vi "ConvertGoop2ToGoop3.vi"() -> (0 "error out":errorcluster)   [LabVIEW 2014]
uses:
  <resource>/Framework/Providers/Open_GDS/ClassProviders/Common/ConvertGoop2ToGoop3_SubVIs/ConvertGoop2ToGoop3_ClassInfo.ctl
  <resource>/Framework/Providers/Open_GDS/ClassProviders/Common/LvClass_class/GDSLvCLass_ClassSettingsType.ctl
  <resource>/Framework/Providers/Open_GDS/ClassProviders/Common/LvClass_class/GDSLvClass_PlugIn.ctl
  <resource>/Framework/Providers/Open_GDS/ClassProviders/Common/LvClass_class/GDSLvClass_PlugInTypes.ctl
  <vilib>/Utility/miscctls.llb/LVPositionTypeDef.ctl
  <vilib>/Utility/error.llb/DialogType.ctl
  <vilib>/picture/picture.llb/imagedata.ctl
  <resource>/Framework/Providers/Open_GDS/ClassProviders/Provider_EndevoGOOP300/Templates/EndevoTemplateNames.ctl
  <resource>/Framework/Providers/Open_GDS/ClassProviders/Provider_EndevoGOOP300/EndevoProviderName.ctl
  <vilib>/regexp/Match Regular Expression.xnode
panel:
  in  "Cancel":bool
  in  "Next":bool
  out "Tab":T1(tab)
  in  "Current GOOP2 top directory":path
  out "Additional VIs that has been found\nand will be relinked:":i32
  out "GOOP2 classes found":string
  in  "VisToRelink":path[](array[path])
  in  "Project":path caption="This project will be created and have all classes added to it:"
  in  "Progress":i32(listbox)
  in  "Done":bool
  out "State":string
  # "1."
  # "Select Top folder to start a recursive search for GOOP2 classes and application VIs."
  # "2."
  # "These classes\nhave been found.\n\nDo you want to convert them?"
  # "3."
  # "Have you backed up all your VIs in the selected folder?"
  # "Have you checked that all files in\nthe selected folder are writeable?"
  # "Relinking VIs outside top folder?\nIf you want to relink any VIs to the new classes that are outside the selected top folder, add them to the list below"
  # "4."
  # "Save VI dialog boxes!?!\nIt might pop up dialog boxes that asks you to save VIs that will be unloaded from memory, JUST press cancel for those."
  # "5."
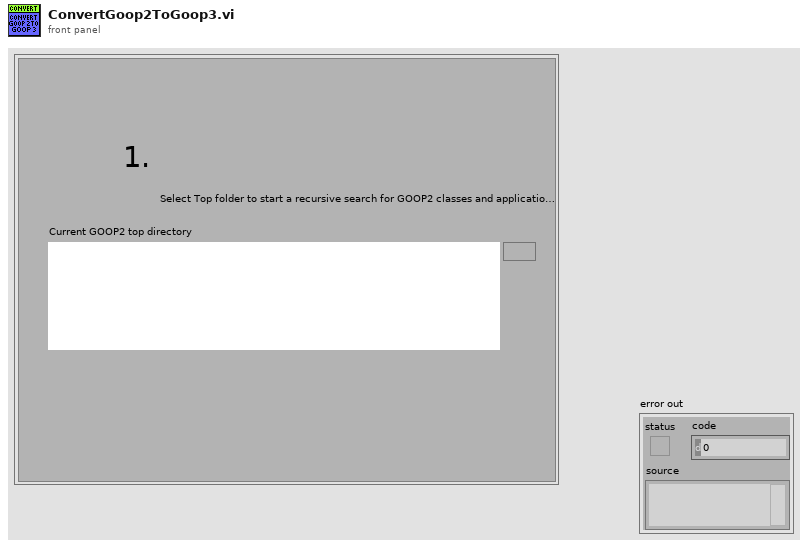
[diagram p1: front panel]
types:
  T1 = enum32{"GOOP2Dir", "ClassesFound", "BackedUp", "Start?", "Converting"}
  T2 = typedef "ConvertGoop2ToGoop3_ClassInfo.ctl" = cluster{"NoOfInheritance":i32, "LvClassPath":path, "ClassName":string, "ClassPrefix":string, "IsLLB":bool, "ClassFolder":path, "ViRefs":refnum<vi>[], "ClassRef":refnum<vi>, "InheritsFrom":path, "RootClass":path, "ViPathes":path[], "AllInheritanceClasses":string[], "TemplateVersionUsed":string, "UsingClassAttributes":bool, "ClassSettings":T3, "HeaderIcon":u8[][]}
  T3 = typedef "GDSLvCLass_ClassSettingsType.ctl" = cluster{"ClassProviderName":string, "ClassTemplateUsed":string, "ClassTemplateVersion":string, "ClassDescription":string, "PlugIns":T4[], "ConnectorPanePattern":string}
  T4 = typedef "GDSLvClass_PlugIn.ctl" = cluster{"Type":T5, "ID":string, "Version":string, "Path":path, "Name":string, "Data":variant}
  T5 = typedef "GDSLvClass_PlugInTypes.ctl" = enum16{"DesignPattern", "MethodTypes"}
  T6 = typedef "LVPositionTypeDef.ctl" = cluster{"Left":i32, "Top":i32}
  T7 = cluster{"TopFolderPath":path, "Classes":T2[], "SetToDynamicDispatch":refnum<vi>[], "error":errorcluster, "Project":path, "ProjectRef":refnum<vi>, "My Computer":refnum<vi>, "AppRef":refnum<vi>, "VIsToRelink":refnum<vi>[], "VIsToRelink(Paths)":path[], "CallParentMethod":cluster{"VIRef":refnum<vi>, "Position":T6}[], "TemplateVersionUsed":string}
  T8 = enum32{"GOOP2Dir", "ClassesFound", "GOOP3Dir", "Start?", "Converting"}
  T9 = typedef "imagedata.ctl" = cluster{"image type":i32, "image depth":i32, "image":u8[], "mask":u8[], "colors":u32[], "Rectangle":cluster{"left":i16, "top":i16, "right":i16, "bottom":i16}}
  T10 = typedef "EndevoTemplateNames.ctl" = enum16{"BaseTemplate", "SubTemplate", "BaseTemplate_4x4x4", "SubTemplate_4x4x4", "SingletonTemplate"}
  T11 = typedef "EndevoProviderName.ctl" = enum16{"EndevoGOOP300"}
  T12 = typedef "DialogType.ctl" = u16
  T13 = enum32{"invalid VI type", "Standard VI", "Control VI", "Global VI", "Polymorphic VI", "Configuration VI", "SubSystem", "Facade VI", "Method VI", "Statechart Diagram VI"}
  T14 = enum16{"Invalid Wire Rule", "Required", "Recommended", "Optional", "Dynamic Dispatch"}
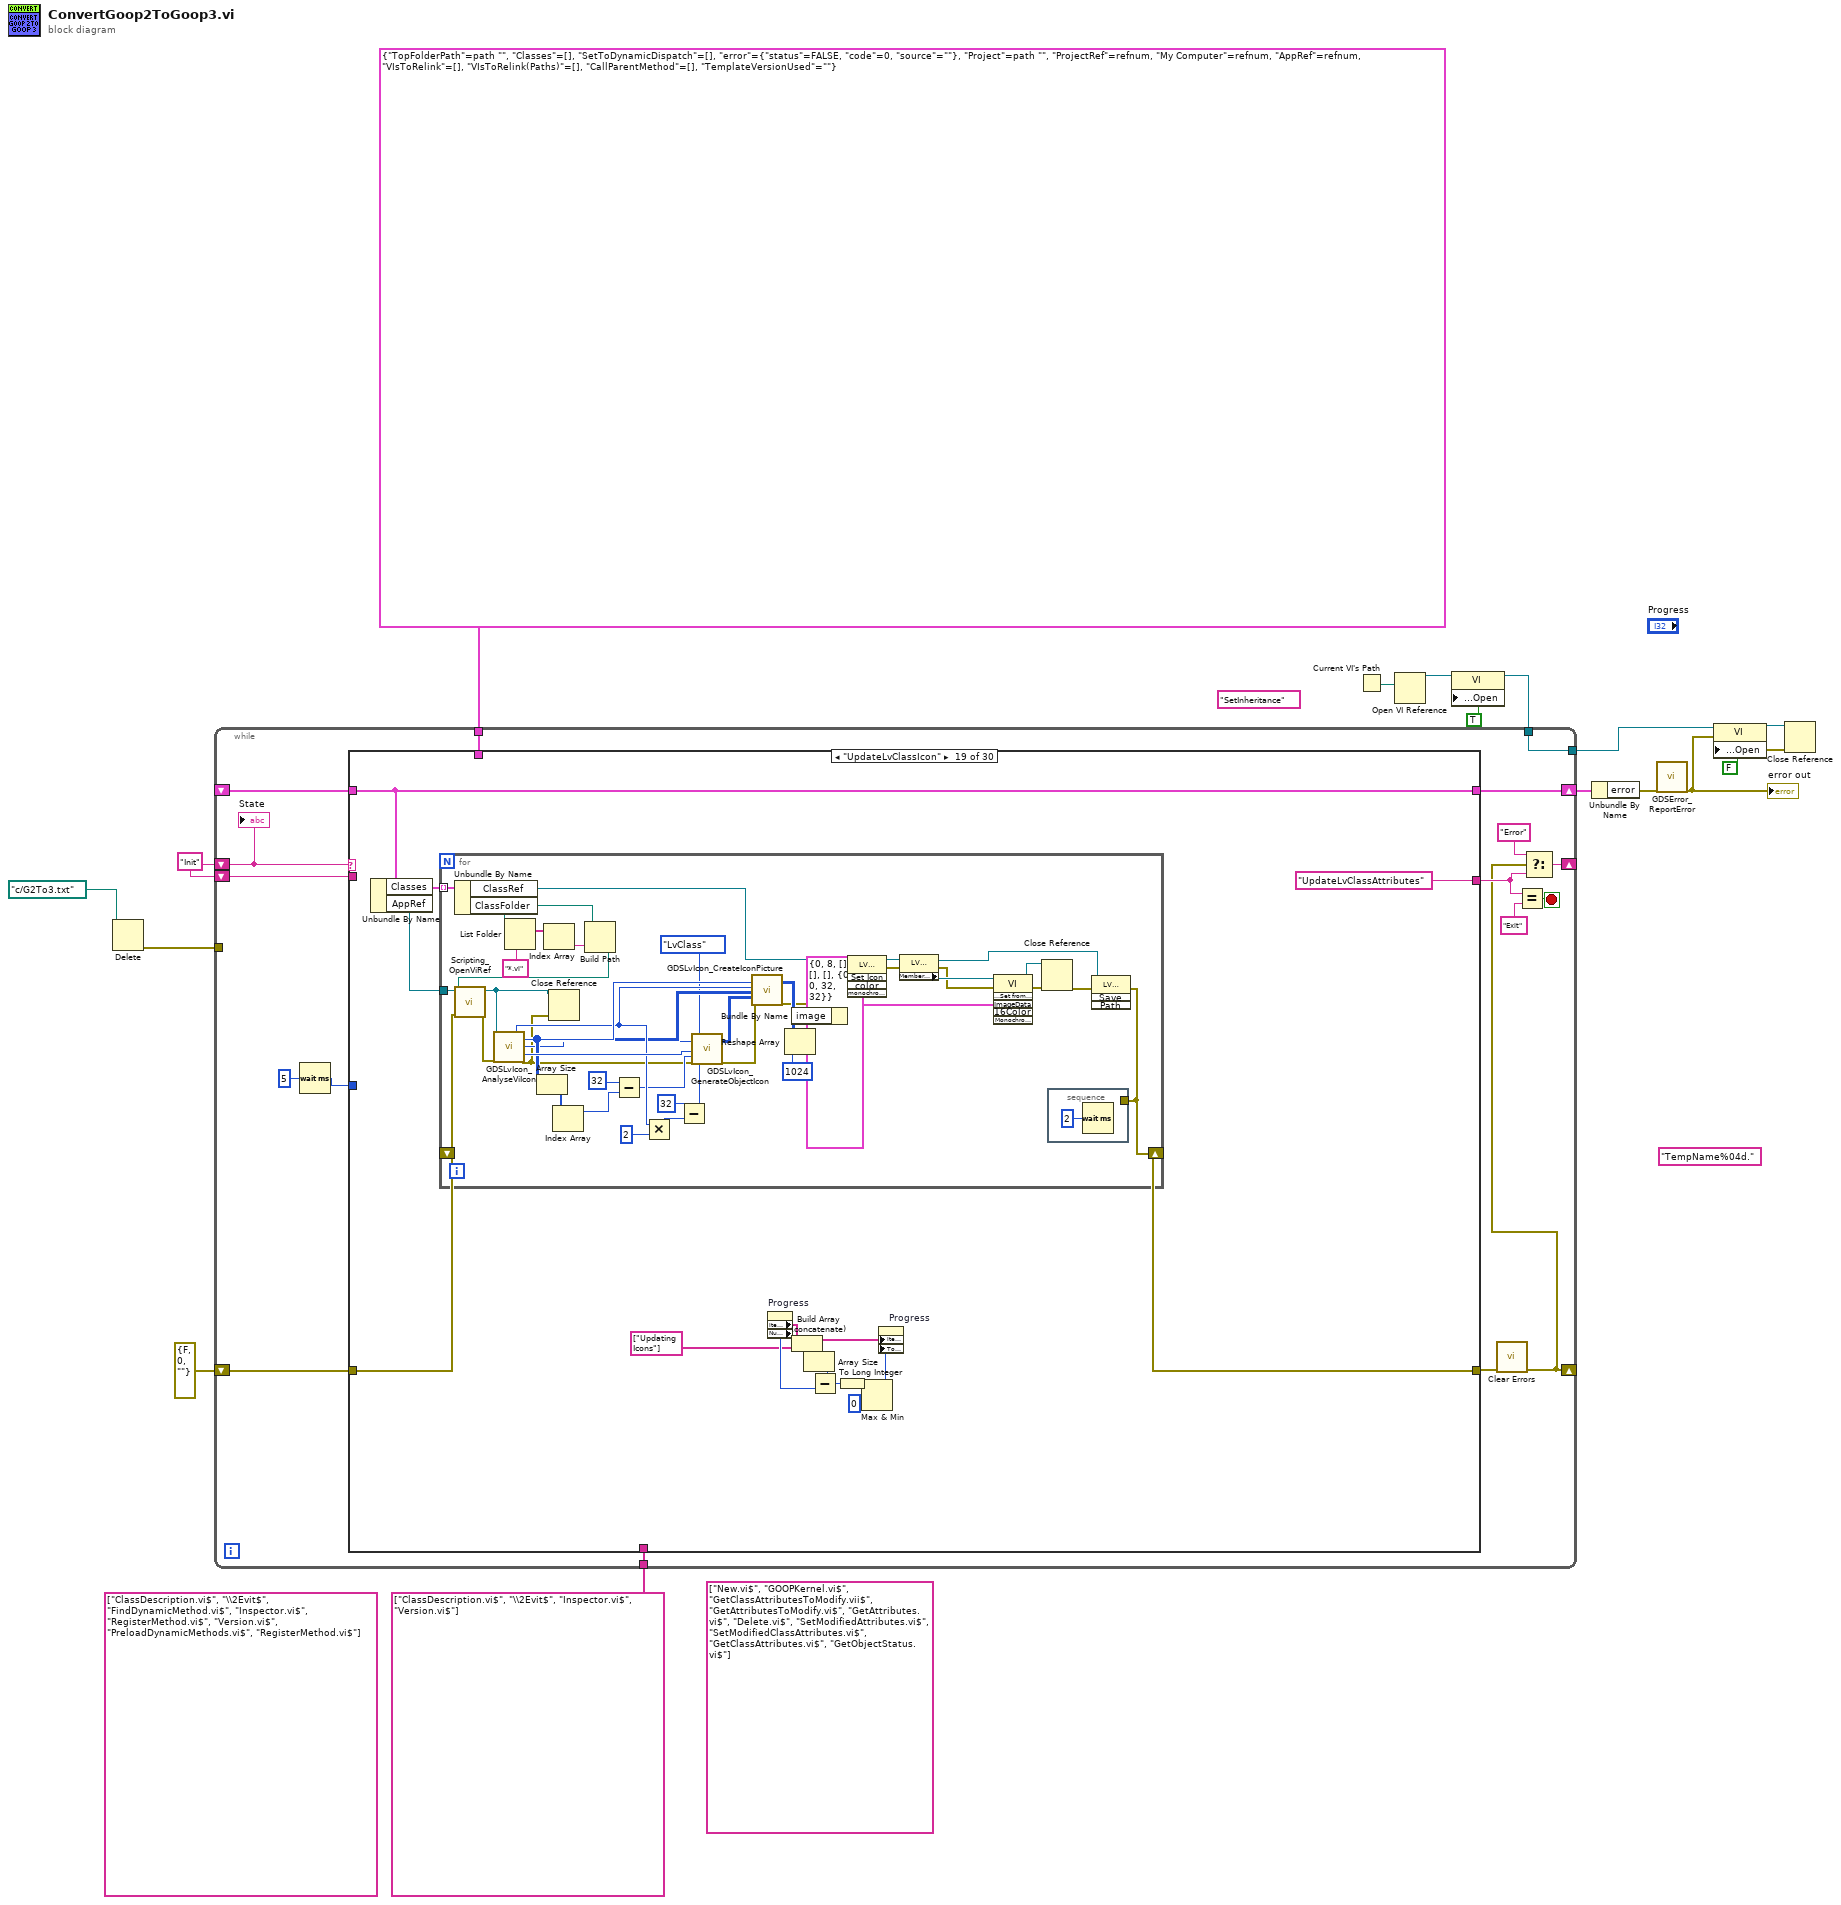
[diagram p0: block diagram]
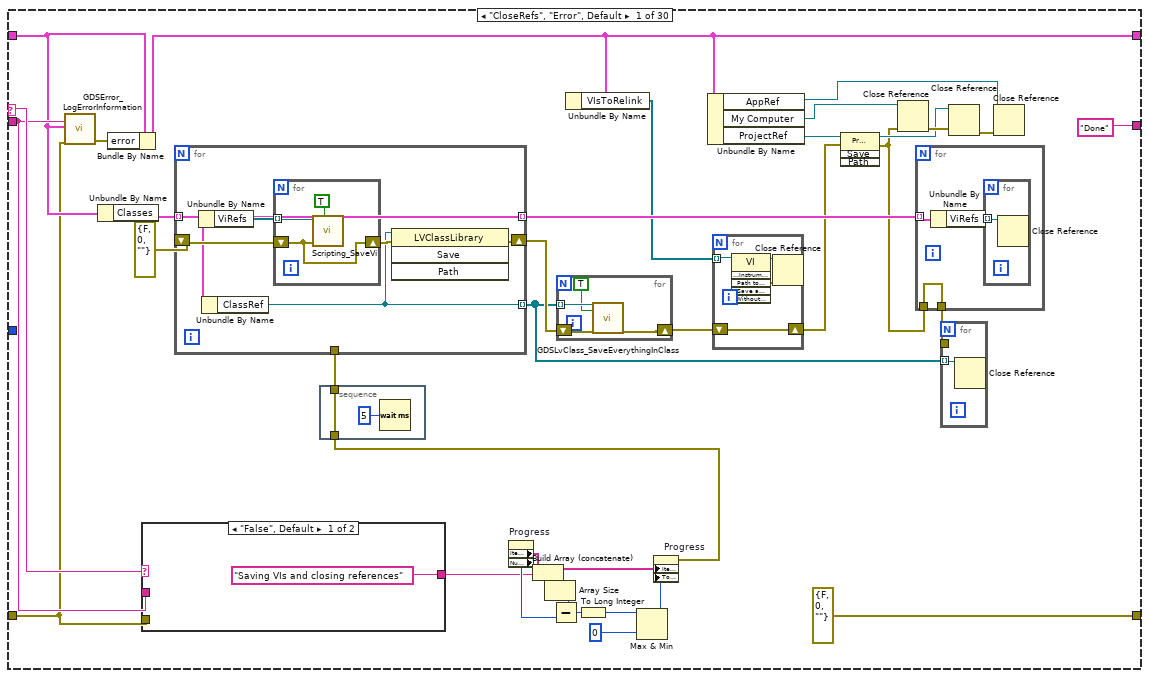
[diagram p2: hidden frame]
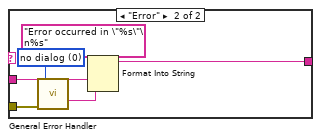
[diagram p3: hidden frame]
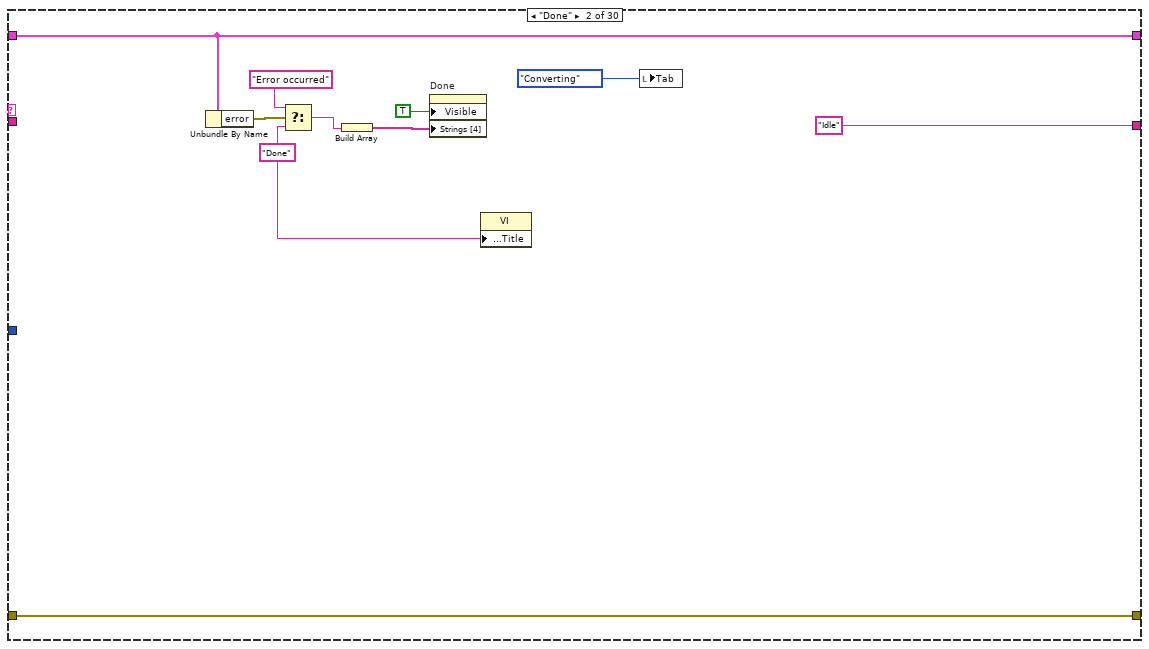
[diagram p4: hidden frame]
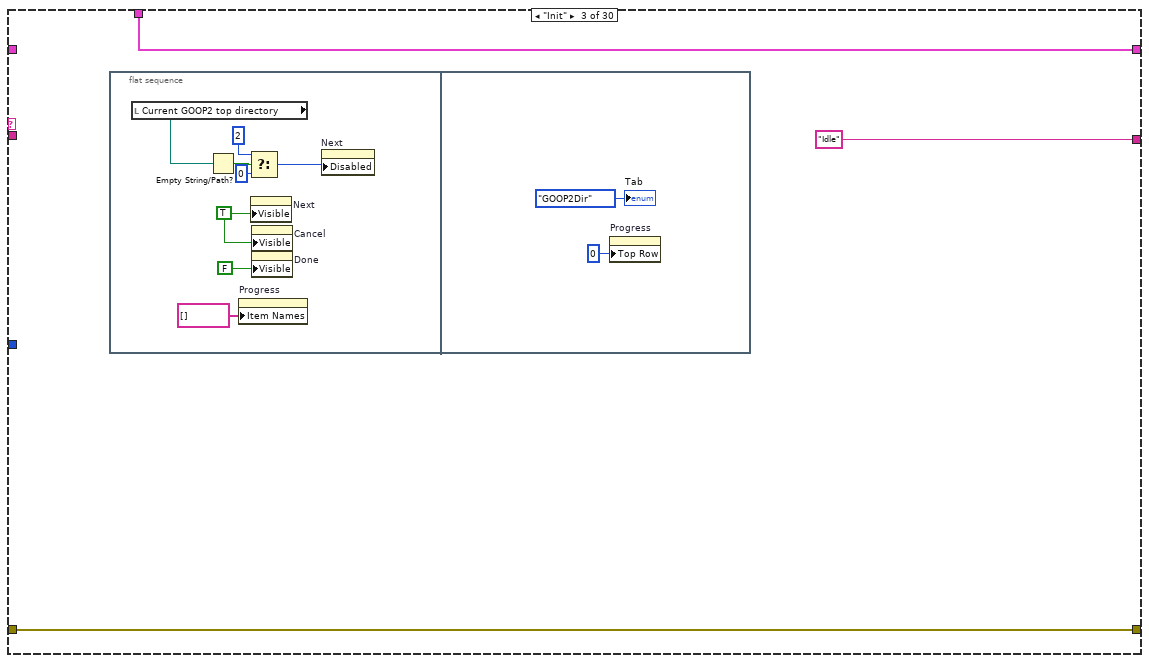
[diagram p5: hidden frame]
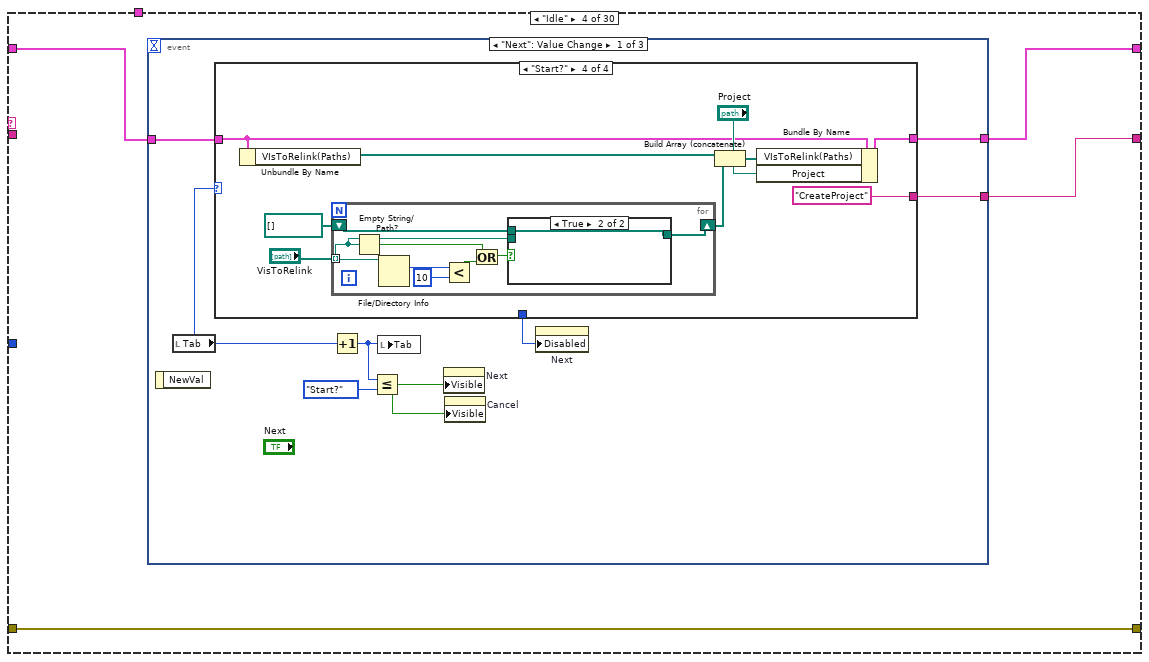
[diagram p6: hidden frame]
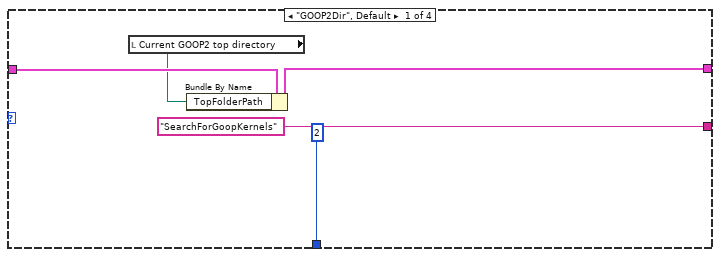
[diagram p7: hidden frame]
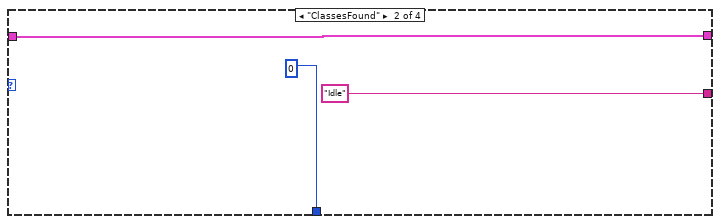
[diagram p8: hidden frame]
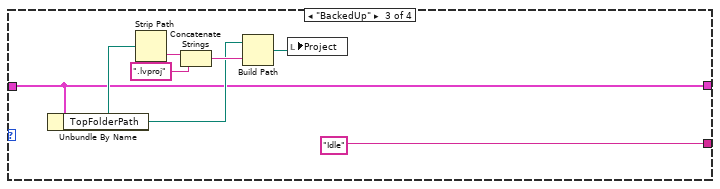
[diagram p9: hidden frame]
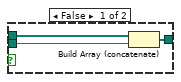
[diagram p10: hidden frame]
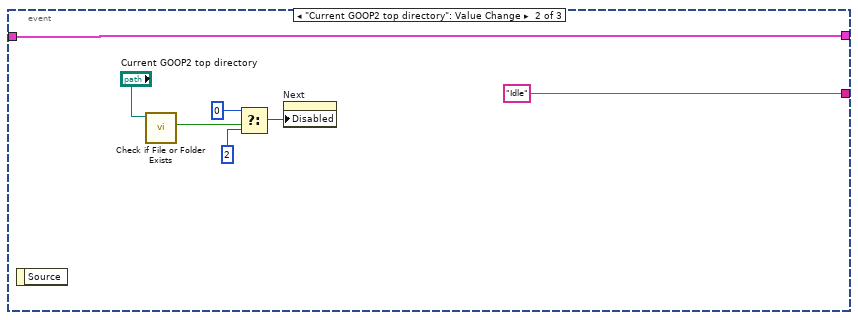
[diagram p11: hidden frame]
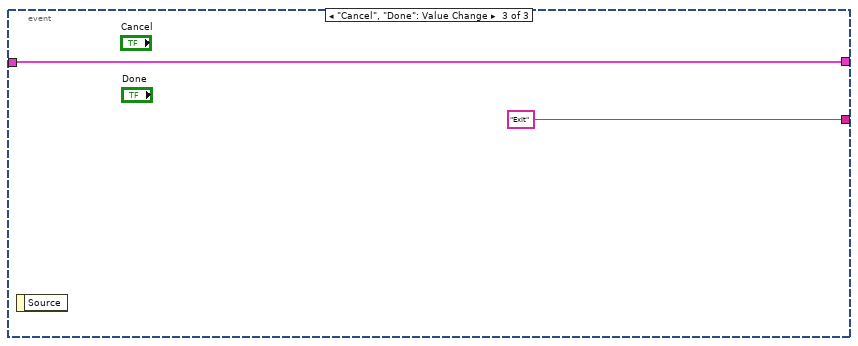
[diagram p12: hidden frame]
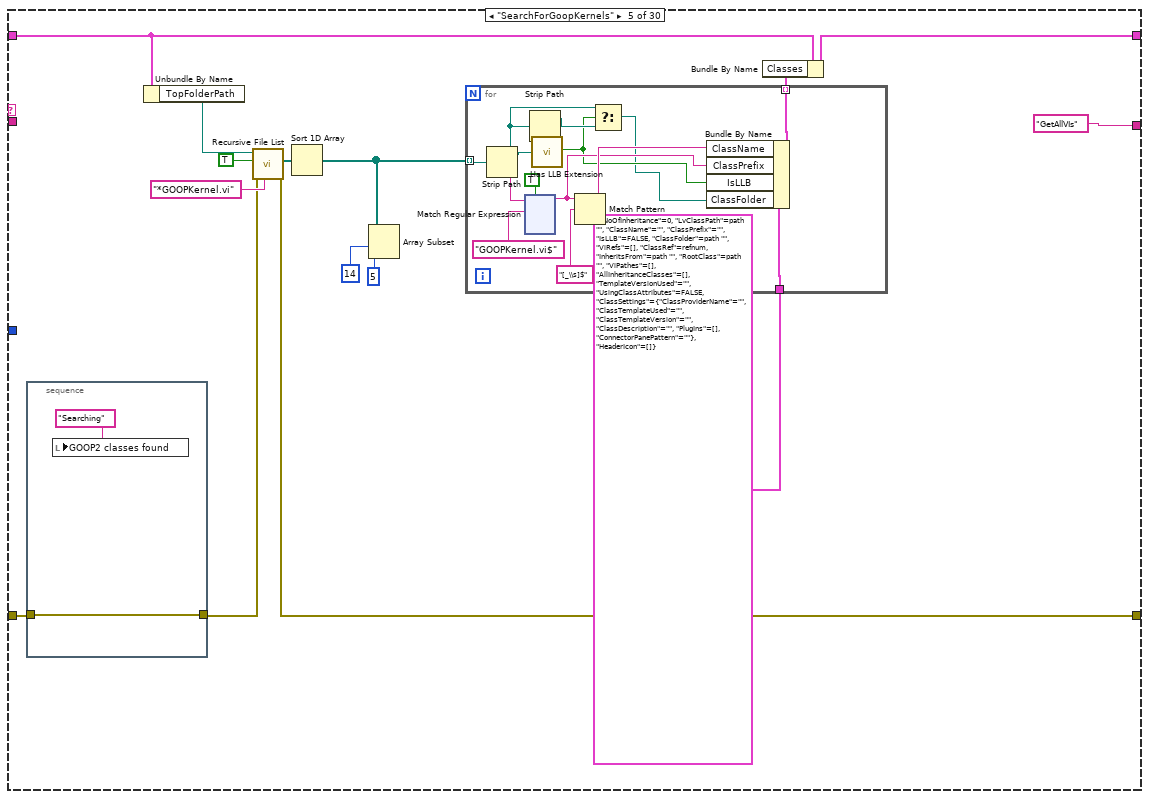
[diagram p13: hidden frame]
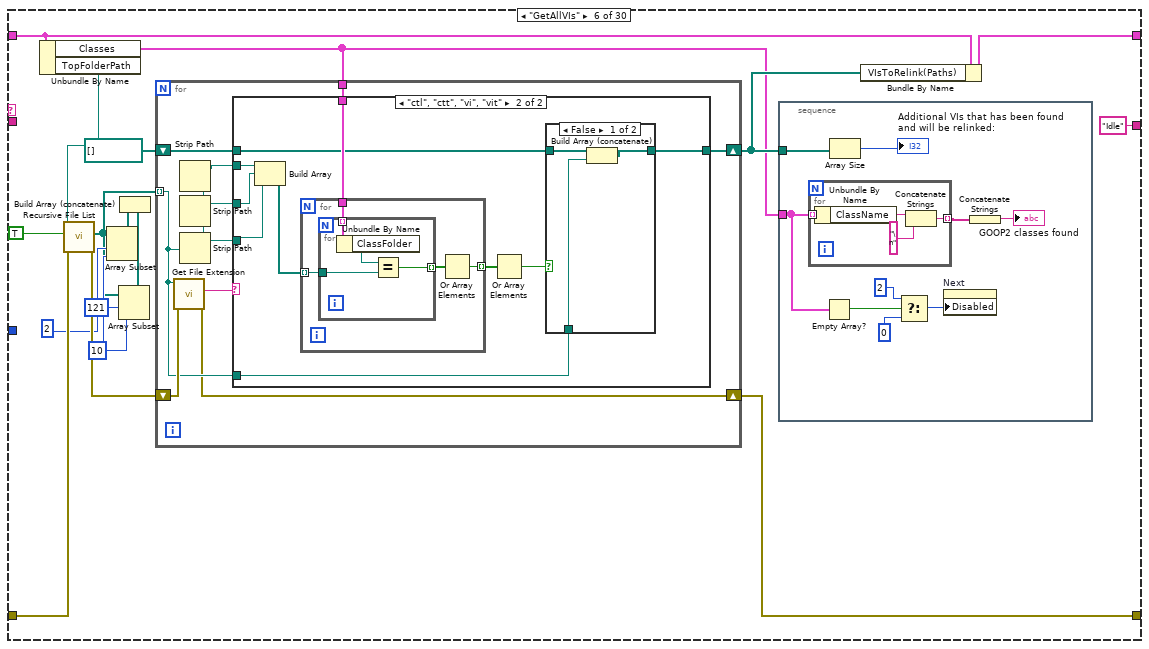
[diagram p14: hidden frame]
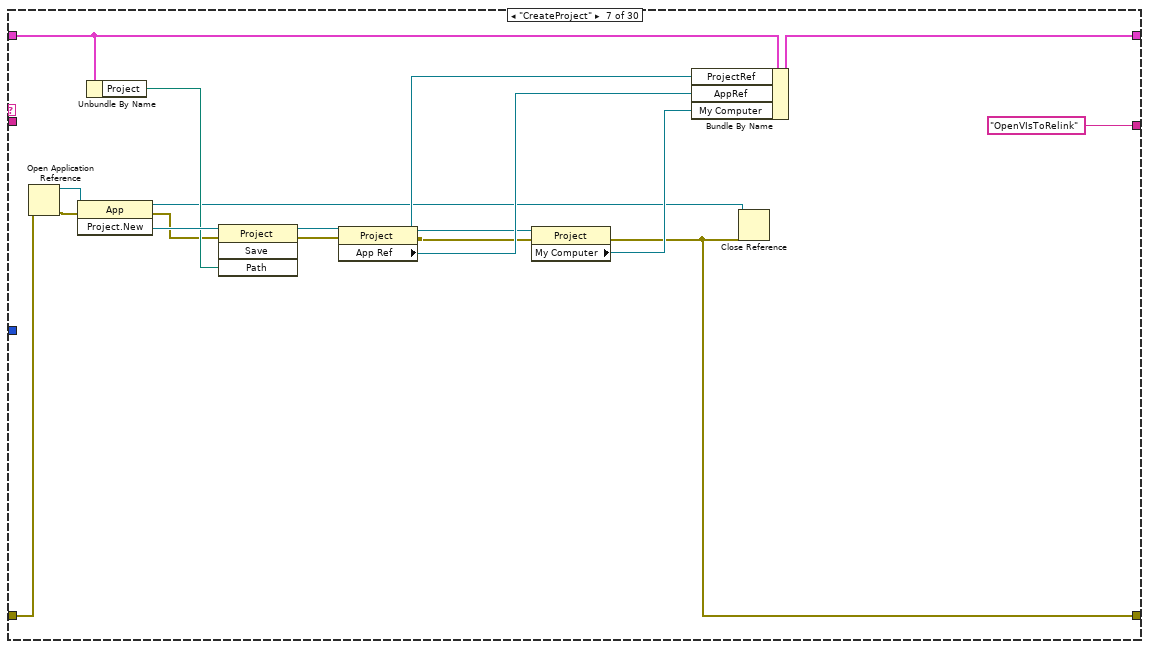
[diagram p17: hidden frame]
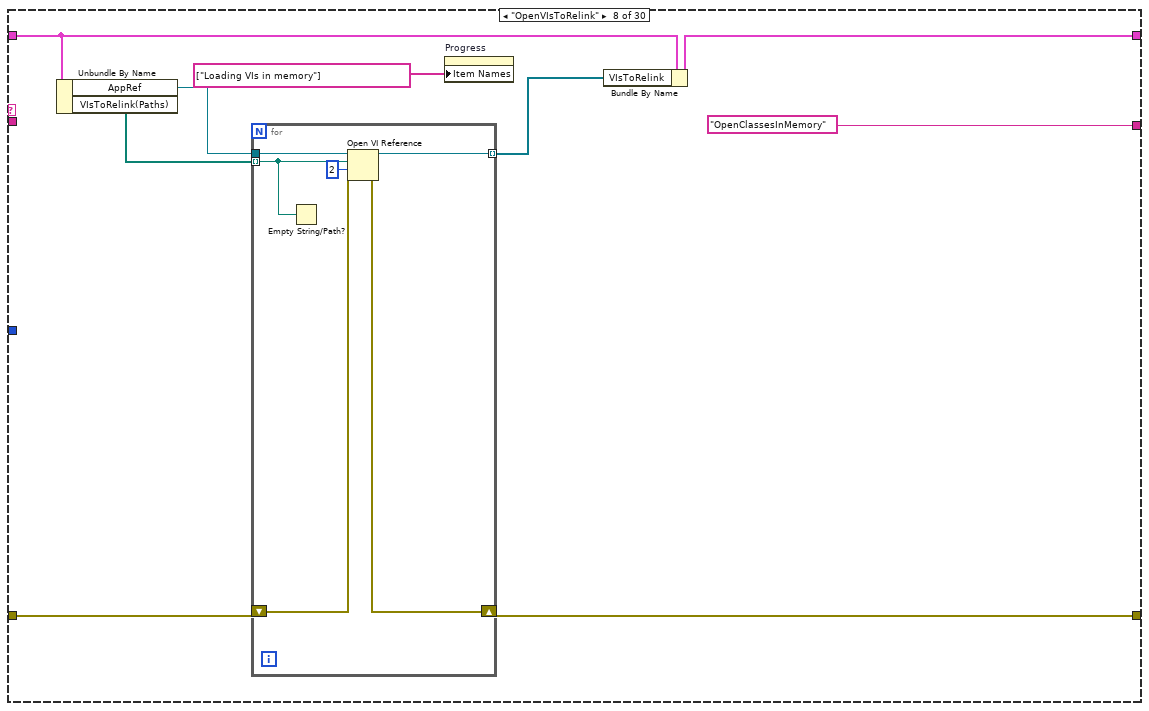
[diagram p18: hidden frame]
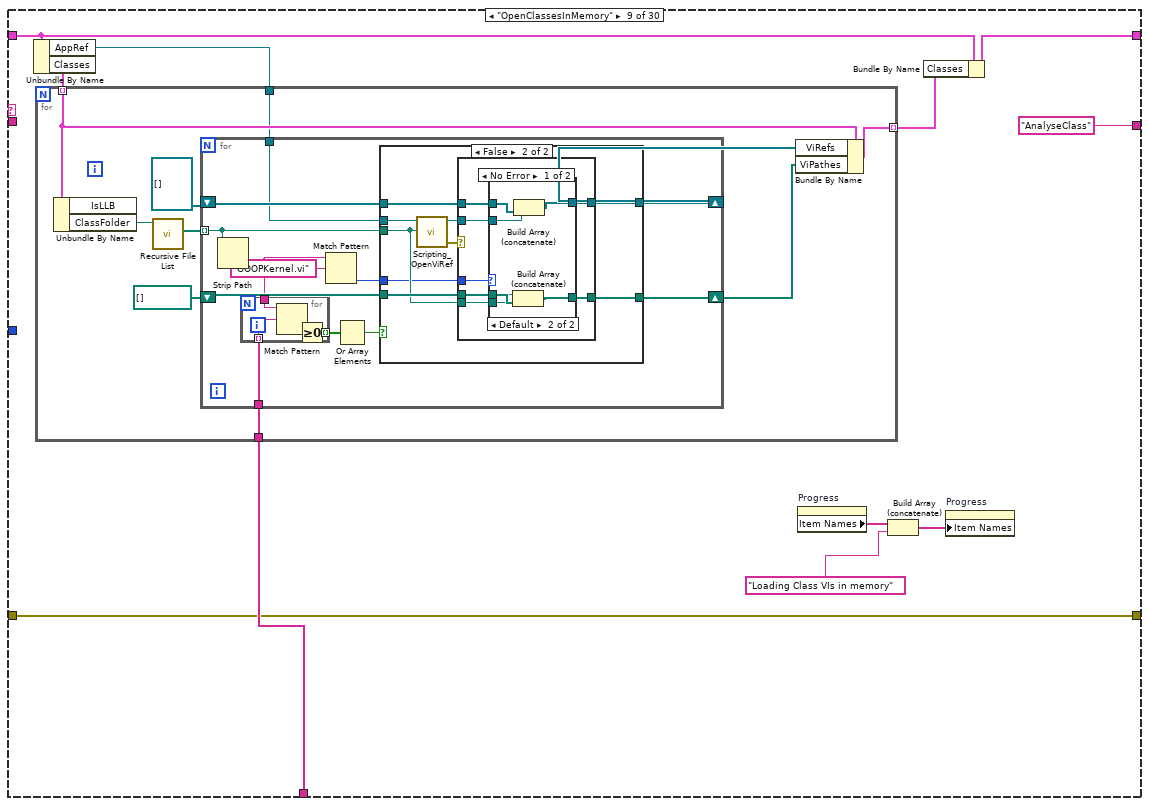
[diagram p19: hidden frame]
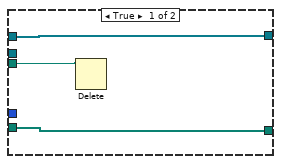
[diagram p20: hidden frame]
diagram:
  (unwired) "SetInheritance"
  (unwired) "TempName%04d." ("format string")
  (unwired) string[] ["ClassDescription.vi$", "\\2Evit$", "FindDynamicMethod.vi$", "Inspector.vi$", "RegisterMethod.vi$", "Version.vi$", "PreloadDynamicMethods.vi$", "RegisterMethod.vi$"] ("file names")
  (unwired) string[] ["New.vi$", "GOOPKernel.vi$", "GetClassAttributesToModify.vii$", "GetAttributesToModify.vi$", "GetAttributes.vi$", "Delete.vi$", "SetModifiedAttributes.vi$", "SetModifiedClassAttributes.vi$", "GetClassAttributes.vi$", "GetObjectStatus.vi$"] ("file names")
  w14 = "Init"
  n1 = Delete(path (use dialog)=path "c:/G2To3.txt" ("file (use dialog)")) -> (error out=w11:errorcluster)  [unwired: 4 in, 2 out]
  n2 = Current VI's Path() -> (path=w9:path)
  n3 = Open VI Reference(vi path=w9) -> (vi reference=w7:refnum<vi>)  [unwired: 5 in, 1 out]
  n4 = property class="VI"(reference=w7, "Front Panel.Open"=TRUE ("Front Panel Window:Open")) -> (reference out=w6:refnum<vi>)  [unwired: 1 in, 1 out]
  n5 = while {
    shift-right: [w18] -> _
    shift-left: errorcluster {"status"=FALSE, "code"=0, "source"=""} ("error IO") -> [w34]
    shift-right: [w33] -> _
    shift-left: w14 -> [w23]
    shift-right: [w28] -> w13
    shift-left: _ -> [w27]
    tunnel: T7 {"TopFolderPath"=path "", "Classes"=[], "SetToDynamicDispatch"=[], "error"={"status"=FALSE, "code"=0, "source"=""}, "Project"=path "", "ProjectRef"=refnum, "My Computer"=refnum, "AppRef"=refnum, "VIsToRelink"=[], "VIsToRelink(Paths)"=[], "CallParentMethod"=[], "TemplateVersionUsed"=""} -> [w26]
    tunnel: string[] ["ClassDescription.vi$", "\\2Evit$", "Inspector.vi$", "Version.vi$"] ("file names") -> [w25]
    shift-left: w14 -> [w24]
    tunnel: w11 -> [_]
    tunnel: w6 -> [w20]
    tunnel: [w20] -> w4
    stop <- w32 stop-if-true
    n6 = Wait (ms)(milliseconds to wait=u32 5) -> (millisecond timer value=w21:u32)
    n7 = case shown="\"UpdateLvClassIcon\"" w23 {
      selector: w23 -> [w64 _ _ _ _ _ _ _ _ _ _ _ _ _ _ _ _ _ _ _ _ _ _ _ _ _ _ _ _ _]
      tunnel: w34 -> [w58 w109 w112 w124 w188 w335 w395 w407 w422 w496 w525 w568 w578 w617 w749 w791 w875 w921 w973 w1022 w1063 w1150 w1212 w1269 w1321 w1401 w1415 w1473 w1507 w1551]
      tunnel: [errorcluster {"status"=FALSE, "code"=0, "source"=""} ("error IO") w109 w112 w124 w192 w333 w386 w406 w422 w496 w524 w566 w574 w618 w752 w790 w886 w923 w974 w1024 w1057 w1137 w1205 w1266 w1327 w1400 w1415 w1474 w1502 w1539] -> w19
      tunnel: ["Done" "Idle" "Idle" w125 "GetAllVIs" "Idle" "OpenVIsToRelink" "OpenClassesInMemory" "AnalyseClass" "RemoveReentrantForDynamicDispatchVIs" "RecompilingVIs" "AddVIsToProject" "RenameFiles" "RenameTempNames" "FindAllCallParentMethodCalls" "UpdateNewVI" "SetInheritance" "UpdateLvClassIcon" "UpdateLvClassAttributes" "UpdateUtilsVIs" "UpdateSubClassKernels" "UpdateVIsGoopRefs" "UpdateCreate" "UpdateDynamicDispatchVIs" "ExtraSave" "SetDynamicDispatch" "UpdateAllCallParentMethods" "UpdateDestroy" "UpdateClassInfo" "CloseRefs"] -> w29
      tunnel: [w47 w108 w111 w126 w190 w331 w397 w409 w425 w494 w526 w567 w571 w616 w750 w788 w873 w922 w976 w1023 w1059 w1136 w1204 w1263 w1324 w1399 w1414 w1471 w1506 w1550] -> w28
      tunnel: w27 -> [w60 w108 _ w127 w191 w332 w399 w410 w426 w495 w526 w567 w571 w611 w750 w789 w873 w922 w976 w1023 w1056 w1136 w1204 w1263 w1319 w1399 w1414 w1471 w1506 w1550]
      tunnel: w26 -> [_ _ w111 _ _ _ _ _ _ _ _ _ _ _ _ _ _ _ _ _ _ _ _ _ _ _ _ _ _ _]
      tunnel: w25 -> [_ _ _ _ _ _ _ _ w423 _ _ _ _ _ _ _ _ _ _ _ _ _ _ _ _ _ _ _ _ _]
      tunnel: w24 -> [w63 _ _ _ _ _ _ _ _ _ _ _ _ _ _ _ _ _ _ _ _ _ _ _ _ _ _ _ _ _]
      tunnel: w21 -> [_ _ _ _ _ _ _ _ _ _ _ _ _ _ _ _ _ _ _ _ _ _ _ _ _ _ _ _ _ _]
      frame "CloseRefs", "Error", Default {
        n8 = call <resource>:"GDSError_LogErrorInformation.vi"("State"=w63, "LocalVariableData"=w60, "error in (no error)"=w58) -> ("error out"=w50:errorcluster)  [unwired: 16 in]
        n9 = Unbundle By Name(w60) -> ("Classes"=w68:T2[])
        n10 = Bundle By Name(cluster=w60, "error"=w50) -> (w47:T7)
        n11 = case shown="\"False\", Default" w64 {
          tunnel: w63 -> [_ w81]
          tunnel: w58 -> [_ w79]
          tunnel: ["Saving VIs and closing references" w77] -> w37
          frame "False", Default {
          }
          frame "Error" {
            w80 = T12 0 items=["no dialog", "OK message", "continue or stop message", "OK message + warnings", "continue/stop + warnings"] ("type of dialog (OK msg:1)")
            n12 = call <vilib>:"General Error Handler.vi"("type of dialog (OK msg:1)"=w80, "error in (no error)"=w79) -> ("message"=w78:string)  [unwired: 9 in, 4 out]
            n13 = Format Into String(format string="Error occurred in \"%s\"\n%s", w81, w78) -> (resulting string=w77:string)  [unwired: 2 in, 1 out]
          }
        }
        n14 = property on="Progress" class="LstBox (strict)"() -> ("Item Names"=w45:string[], "Number of Rows"=w39:u32)  [unwired: 2 in, 2 out]
        n15 = Build Array (concatenate)(w45, w37) -> (w40:string[])
        n16 = Array Size(array=w40) -> (size(s)=w44:i32)
        n17 = Subtract(x=w44, y=w39) -> (x-y=w43:u32)
        n18 = Unbundle By Name(w47) -> ("VIsToRelink"=w52:refnum<vi>[])
        n19 = To Long Integer(number=w43) -> (32bit integer=w41:i32)
        n20 = Max & Min(x=w41, y=0) -> (max(x,y)=w38:i32)  [unwired: 1 out]
        n21 = property on="Progress" class="LstBox (strict)"("Item Names"=w40, "Top Row"=w38) -> (error out=w36:errorcluster)  [unwired: 2 in, 1 out]
        n22 = stacked-sequence {
          tunnel: w36 -> [w70]
          tunnel: [w70] -> w35
          frame #0 {
            n23 = Wait (ms)(milliseconds to wait=u32 5) -> ()  [unwired: 1 out]
          }
        }
        n24 = for {
          tunnel: w68 -> [w95] mode=indexing
          tunnel: [w95] -> w67 mode=indexing
          shift-right: [w93] -> w66
          shift-left: errorcluster {"status"=FALSE, "code"=0, "source"=""} ("error out") -> [w96]
          tunnel: [w92] -> w65 mode=indexing
          tunnel: w35 -> [_]
          n25 = Unbundle By Name(w95) -> ("ViRefs"=w97:refnum<vi>[])
          n26 = Unbundle By Name(w95) -> ("ClassRef"=w92:refnum<vi>)
          n27 = for {
            tunnel: w97 -> [w100] mode=indexing
            shift-right: [w98] -> w94
            shift-left: w96 -> [w98]
            n28 = call <resource>:"Scripting_SaveVi.vi"("ForceResaving(False)"=TRUE, "error in (no error)"=w98, "VIRefToSaveIn"=w100) -> ()  [unwired: 7 in, 2 out]
          }
          n29 = invoke class="LVClassLibrary" method="Save"(reference=w92, error in=w94) -> (error out=w93:errorcluster)  [unwired: 2 in, 3 out]
        }
        n30 = for {
          shift-right: [w86] -> w49
          shift-left: w66 -> [w87]
          tunnel: w65 -> [w85] mode=indexing
          n31 = call <resource>:"GDSLvClass_SaveEverythingInClass.vi"("ClassRefIn"=w85, "ForceResaving(False)"=TRUE, "error in"=w87) -> ("error out"=w86:errorcluster)  [unwired: 15 in, 1 out]
        }
        n32 = Unbundle By Name(w47) -> ("AppRef"=w53:refnum<vi>, "My Computer"=w46:refnum<vi>, "ProjectRef"=w57:refnum<vi>)
        n33 = for {
          tunnel: w52 -> [w73] mode=indexing
          shift-right: [w72] -> w48
          shift-left: w49 -> [w72]
          n34 = invoke class="VI" method="Save.Instrument"(reference=w73) -> (reference out=w74:refnum<vi>, error out=w75:errorcluster)  [unwired: 5 in, 4 out]
          n35 = Close Reference(reference=w74, error in (no error)=w75) -> ()  [unwired: 1 out]
        }
        n36 = invoke class="Project" method="Save"(reference=w57, error in=w48) -> (reference out=w55:refnum<vi>, error out=w51:errorcluster)  [unwired: 2 in, 2 out]
        n37 = Close Reference(reference=w46, error in (no error)=w51) -> (error out=w56:errorcluster)
        n38 = for {
          tunnel: w67 -> [w90] mode=indexing
          tunnel: w51 -> [w88]
          tunnel: [w88] -> w62
          n39 = Unbundle By Name(w90) -> ("ViRefs"=w89:refnum<vi>[])
          n40 = for {
            tunnel: w89 -> [w91] mode=indexing
            n41 = Close Reference(reference=w91) -> ()  [unwired: 1 in, 1 out]
          }
        }
        n42 = for {
          tunnel: w65 -> [w83] mode=indexing
          tunnel: w62 -> [_]
          n43 = Close Reference(reference=w83) -> ()  [unwired: 1 in, 1 out]
        }
        n44 = Close Reference(reference=w55, error in (no error)=w56) -> (error out=w54:errorcluster)
        n45 = Close Reference(reference=w53, error in (no error)=w54) -> ()  [unwired: 1 out]
      }
      frame "Done" {
        w101 = "Done"
        n46 = Unbundle By Name(w108) -> ("error"=w107:errorcluster)
        n47 = Select(t="Error occurred", s=w107, f=w101) -> (s? t:f=w104:string)
        n48 = Build Array(w104) -> (w103:string[])
        n49 = property on="Done" class="Bool"("Visible"=TRUE, "Strings [4]"=w103) -> ()  [unwired: 2 in, 2 out]
        n50 = property class="VI"("Front Panel.Title"=w101) -> ()  [unwired: 2 in, 2 out]
        n51 = local write "Tab"(T1."Converting" ("Tab")) -> ()
      }
      frame "Init" {
        n52 = flat-sequence {
          frame #0 {
            w121 = TRUE ("Visible")
            n53 = local read "Current GOOP2 top directory"() -> (w118:path)
            n54 = Empty String/Path?(string/path=w118) -> (empty?=w117:bool)
            n55 = property on="Progress" class="LstBox (strict)"("Item Names"=string[] []) -> ()  [unwired: 2 in, 2 out]
            n56 = Select(t=u8 2 ("Disabled"), s=w117, f=u8 0) -> (s? t:f=w115:u8)
            n57 = property on="Next" class="Bool"("Visible"=w121) -> ()  [unwired: 2 in, 2 out]
            n58 = property on="Cancel" class="Bool"("Visible"=w121) -> ()  [unwired: 2 in, 2 out]
            n59 = property on="Done" class="Bool"("Visible"=FALSE) -> ()  [unwired: 2 in, 2 out]
            n60 = property on="Next" class="Bool"("Disabled"=w115) -> ()  [unwired: 2 in, 2 out]
          }
          frame #1 {
            n61 = property on="Progress" class="LstBox (strict)"("Top Row"=0) -> ()  [unwired: 2 in, 2 out]
            "Tab" <- T1."GOOP2Dir" ("Tab")
          }
        }
      }
      frame "Idle" {
        n62 = event shown="[0] \"Next\": Value Change" {
          selector: _ -> [_ _ _]
          dyn-events: _ -> [_ _ _]
          timeout: _ -> [_ _ _]
          tunnel: w127 -> [w131 w174 w179]
          tunnel: [w130 w174 w179] -> w126
          tunnel: [w129 "Idle" "Exit"] -> w125
          event "Next": Value Change {
            n63 = event-data() -> ()  [unwired: 1 in, 1 out]
            n64 = local read "Tab"() -> (w132:T1)
            n65 = case shown="\"Start?\"" w132 {
              tunnel: w131 -> [w140 w142 w145 w156]
              tunnel: [w139 w142 w145 w159] -> w130
              tunnel: ["SearchForGoopKernels" "Idle" "Idle" "CreateProject"] -> w129
              tunnel: [u8 2 ("Disabled") u8 0 ("f") _ _] -> w128
              frame "GOOP2Dir", Default {
                n66 = local read "Current GOOP2 top directory"() -> (w137:path)
                n67 = Bundle By Name(cluster=w140, "TopFolderPath"=w137) -> (w139:T7)
              }
              frame "ClassesFound" {
              }
              frame "BackedUp" {
                n68 = Unbundle By Name(w145) -> ("TopFolderPath"=w146:path)
                n69 = Strip Path(path=w146) -> (name=w149:string)  [unwired: 1 out]
                n70 = Concatenate Strings(w149, ".lvproj" ("string")) -> (w147:string)
                n71 = Build Path(base path=w146, name or relative path=w147) -> (appended path=w144:path)
                n72 = local write "Project"(w144) -> ()
              }
              frame "Start?" {
                n73 = Unbundle By Name(w156) -> ("VIsToRelink(Paths)"=w155:path[])
                n74 = for {
                  tunnel: "VisToRelink" -> [w161] mode=indexing
                  shift-right: [w160] -> w151
                  shift-left: path[] [] -> [w162]
                  n75 = Empty String/Path?(string/path=w161) -> (empty?=w164:bool)
                  n76 = File/Directory Info(path=w161) -> (size=w167:i64)  [unwired: 1 in, 6 out]
                  n77 = Less?(x=w167, y=i64 10) -> (x < y?=w165:bool)
                  n78 = Or(x=w164, y=w165) -> (x .or. y?=w163:bool)
                  n79 = case shown="True" w163 {
                    tunnel: w162 -> [w170 w171]
                    tunnel: w161 -> [w169 _]
                    tunnel: [w168 w171] -> w160
                    frame False {
                      n80 = Build Array (concatenate)(w170, w169) -> (w168:path[])
                    }
                    frame True {
                    }
                  }
                }
                n81 = Build Array (concatenate)(w155, w151) -> (w154:path[])
                n82 = Bundle By Name(cluster=w156, "VIsToRelink(Paths)"=w154, "Project"="Project") -> (w159:T7)
              }
            }
            n83 = Increment(x=w132) -> (x+1=w135:T1)
            n84 = Less Or Equal?(x=w135, y=T8."Start?") -> (x <= y?=w133:bool)
            n85 = local write "Tab"(w135) -> ()
            n86 = property on="Next" class="Bool"("Visible"=w133) -> ()  [unwired: 2 in, 2 out]
            n87 = property on="Cancel" class="Bool"("Visible"=w133) -> ()  [unwired: 2 in, 2 out]
            n88 = property on="Next" class="Bool"("Disabled"=w128) -> ()  [unwired: 2 in, 2 out]
          }
          event "Current GOOP2 top directory": Value Change {
            n89 = event-data() -> ()  [unwired: 1 in, 1 out]
            n90 = call <vilib>:"Check if File or Folder Exists.vi"("path"="Current GOOP2 top directory") -> ("file or folder exists?"=w178:bool)  [unwired: 8 in, 2 out]
            n91 = Select(t=u8 0, s=w178, f=u8 2 ("Disabled")) -> (s? t:f=w177:u8)
            n92 = property on="Next" class="Bool"("Disabled"=w177) -> ()  [unwired: 2 in, 2 out]
          }
          event "Cancel", "Done": Value Change {
            n93 = event-data() -> ()  [unwired: 1 in, 1 out]
          }
        }
      }
      frame "SearchForGoopKernels" {
        n94 = stacked-sequence {
          tunnel: w188 -> [w196]
          tunnel: [w196] -> w187
          frame #0 {
            n95 = local write "GOOP2 classes found"("Searching" ("GOOP2 classes found")) -> ()
          }
        }
        n96 = Unbundle By Name(w191) -> ("TopFolderPath"=w195:path)
        n97 = call <vilib>:"Recursive File List.vi"("pattern"="*GOOPKernel.vi", "error in (no error)"=w187, "Treat LLBs as Folders?"=TRUE, "Folder Path"=w195) -> ("error out"=w192:errorcluster, "All Files in Dir"=w186:path[])  [unwired: 3 in, 3 out]
        n98 = Sort 1D Array(array=w186) -> (sorted array=w182:path[])
        n99 = Array Subset(array=w182, index=14, length=5) -> ()  [unwired: 1 out]
        n100 = for {
          tunnel: w182 -> [w210] mode=indexing
          tunnel: T2 {"NoOfInheritance"=0, "LvClassPath"=path "", "ClassName"="", "ClassPrefix"="", "IsLLB"=FALSE, "ClassFolder"=path "", "ViRefs"=[], "ClassRef"=refnum, "InheritsFrom"=path "", "RootClass"=path "", "ViPathes"=[], "AllInheritanceClasses"=[], "TemplateVersionUsed"="", "UsingClassAttributes"=FALSE, "ClassSettings"={"ClassProviderName"="", "ClassTemplateUsed"="", "ClassTemplateVersion"="", "ClassDescription"="", "PlugIns"=[], "ConnectorPanePattern"=""}, "HeaderIcon"=[]} ("output cluster") -> [w203]
          tunnel: [w198] -> w181 mode=indexing
          n101 = Strip Path(path=w210) -> (stripped path=w205:path, name=w209:string)
          n102 = xnode "Match Regular Expression"("input string"=w209, "regular expression"="GOOPKernel.vi$", "ignore case? (F)"=TRUE) -> ("before match"=w201:string)  [unwired: 3 in, 4 out]
          n103 = Strip Path(path=w205) -> (stripped path=w204:path)  [unwired: 1 out]
          n104 = call <vilib>:"Has LLB Extension.vi"("path"=w205) -> ("path to VI library?"=w200:bool)
          n105 = Match Pattern(string=w201, regular expression="[_\\s]$") -> (before substring=w202:string)  [unwired: 1 in, 3 out]
          n106 = Select(t=w205, s=w200, f=w204) -> (s? t:f=w199:path)
          n107 = Bundle By Name(cluster=w203, "ClassName"=w202, "ClassPrefix"=w201, "IsLLB"=w200, "ClassFolder"=w199) -> (w198:T2)
        }
        n108 = Bundle By Name(cluster=w191, "Classes"=w181) -> (w190:T7)
      }
      frame "GetAllVIs" {
        w326 = 10 ("length")
        n109 = Unbundle By Name(w332) -> ("Classes"=w329:T2[], "TopFolderPath"=w338:path)
        n110 = call <vilib>:"Recursive File List.vi"("error in (no error)"=w335, "Treat LLBs as Folders?"=TRUE, "Folder Path"=w338) -> ("error out"=w334:errorcluster, "All Files in Dir"=w322:path[])  [unwired: 4 in, 3 out]
        n111 = Array Subset(array=w322, index=2, length=w326) -> (w324:path[])
        n112 = Array Subset(array=w322, index=121, length=w326) -> (w323:path[])
        n113 = Build Array (concatenate)(w324, w323) -> ()  [unwired: 1 out]
        n114 = for {
          shift-right: [w360] -> w330
          shift-left: path[] [] ("All Files in Dir") -> [w359]
          tunnel: w322 -> [w353] mode=indexing
          shift-right: [w352] -> w333
          shift-left: w334 -> [w358]
          tunnel: w329 -> [w354]
          n115 = call <vilib>:"Get File Extension.vi"("error in (no error)"=w358, "file"=w353) -> ("error out"=w352:errorcluster, "lowercase file extension"=w361:string)  [unwired: 6 in, 2 out]
          n116 = Strip Path(path=w353) -> (stripped path=w357:path)  [unwired: 1 out]
          n117 = Strip Path(path=w357) -> (stripped path=w355:path)  [unwired: 1 out]
          n118 = Strip Path(path=w355) -> (stripped path=w356:path)  [unwired: 1 out]
          n119 = case shown="\"ctl\", \"ctt\", \"vi\", \"vit\"" w361 {
            tunnel: [w362 w365] -> w360
            tunnel: w359 -> [w362 w364]
            tunnel: w357 -> [_ w370]
            tunnel: w356 -> [_ w372]
            tunnel: w355 -> [_ w371]
            tunnel: w354 -> [_ w368]
            tunnel: w353 -> [_ w363]
            frame Default {
            }
            frame "ctl", "ctt", "vi", "vit" {
              n120 = Build Array(w372, w371, w370) -> (w369:path[])
              n121 = for {
                tunnel: w369 -> [w379] mode=indexing
                tunnel: w368 -> [w380]
                tunnel: [w377] -> w367 mode=indexing
                n122 = for {
                  tunnel: w380 -> [w384] mode=indexing
                  tunnel: w379 -> [w382]
                  tunnel: [w381] -> w378 mode=indexing
                  n123 = Unbundle By Name(w384) -> ("ClassFolder"=w383:path)
                  n124 = Equal?(x=w383, y=w382) -> (x = y?=w381:bool)
                }
                n125 = Or Array Elements(Boolean array=w378) -> (logical OR=w377:bool)
              }
              n126 = Or Array Elements(Boolean array=w367) -> (logical OR=w366:bool)
              n127 = case shown="False" w366 {
                tunnel: [w374 w376] -> w365
                tunnel: w364 -> [w375 w376]
                tunnel: w363 -> [w373 _]
                frame False {
                  n128 = Build Array (concatenate)(w375, w373) -> (w374:path[])
                }
                frame True {
                }
              }
            }
          }
        }
        n129 = stacked-sequence {
          tunnel: w329 -> [w339]
          tunnel: w330 -> [w341]
          frame #0 {
            n130 = for {
              tunnel: w339 -> [w351] mode=indexing
              tunnel: [w348] -> w347 mode=indexing
              n131 = Unbundle By Name(w351) -> ("ClassName"=w350:string)
              n132 = Concatenate Strings(w350, "\n" ("string")) -> (w348:string)
            }
            n133 = Empty Array?(array=w339) -> (empty?=w342:bool)
            n134 = Array Size(array=w341) -> (size(s)=→"Additional VIs that has been found\nand will be relinked:":i32)
            n135 = Select(t=u8 2, s=w342, f=u8 0 ("Disabled")) -> (s? t:f=w345:u8)
            n136 = property on="Next" class="Bool"("Disabled"=w345) -> ()  [unwired: 2 in, 2 out]
            n137 = Concatenate Strings(w347) -> (→"GOOP2 classes found":string)
          }
        }
        n138 = Bundle By Name(cluster=w332, "VIsToRelink(Paths)"=w330) -> (w331:T7)
      }
      frame "CreateProject" {
        n139 = Open Application Reference(8:w395) -> (0:w396:errorcluster, 3:w394:refnum<vi>)  [unwired: 3 in]
        n140 = invoke class="App" method="Project.New"(reference=w394, error in=w396) -> (reference out=w385:refnum<vi>, error out=w398:errorcluster, "Project:New"=w401:refnum<vi>)  [unwired: 1 in]
        n141 = Unbundle By Name(w399) -> ("Project"=w400:path)
        n142 = invoke class="Project" method="Save"(reference=w401, error in=w398, "Path"=w400) -> (reference out=w390:refnum<vi>, error out=w391:errorcluster)  [unwired: 1 in, 2 out]
        n143 = property class="Project"(reference=w390, error in=w391) -> (reference out=w389:refnum<vi>, error out=w388:errorcluster, "App Ref"=w392:refnum<vi>)
        n144 = property class="Project"(reference=w389, error in=w388) -> (error out=w386:errorcluster, "My Computer"=w387:refnum<vi>)  [unwired: 1 out]
        n145 = Bundle By Name(cluster=w399, "ProjectRef"=w389, "AppRef"=w392, "My Computer"=w387) -> (w397:T7)
        n146 = Close Reference(reference=w385, error in (no error)=w386) -> ()  [unwired: 1 out]
      }
      frame "OpenVIsToRelink" {
        n147 = Unbundle By Name(w410) -> ("AppRef"=w408:refnum<vi>, "VIsToRelink(Paths)"=w402:path[])
        n148 = for {
          tunnel: w408 -> [w416]
          shift-right: [w414] -> w406
          shift-left: w407 -> [w415]
          tunnel: [w413] -> w405 mode=indexing
          tunnel: w402 -> [w411] mode=indexing
          n149 = Empty String/Path?(string/path=w411) -> ()  [unwired: 1 out]
          n150 = Open VI Reference(application reference (local)=w416, vi path=w411, options=2, error in (no error)=w415) -> (vi reference=w413:refnum<vi>, error out=w414:errorcluster)  [unwired: 2 in]
        }
        n151 = property on="Progress" class="LstBox (strict)"("Item Names"=string[] ["Loading VIs in memory"]) -> ()  [unwired: 2 in, 2 out]
        n152 = Bundle By Name(cluster=w410, "VIsToRelink"=w405) -> (w409:T7)
      }
      frame "OpenClassesInMemory" {
        n153 = Unbundle By Name(w426) -> ("AppRef"=w420:refnum<vi>, "Classes"=w427:T2[])
        n154 = for {
          tunnel: w427 -> [w434] mode=indexing
          tunnel: [w432] -> w421 mode=indexing
          tunnel: w423 -> [w431]
          tunnel: w420 -> [w428]
          n155 = Unbundle By Name(w434) -> ("ClassFolder"=w437:path)  [unwired: 1 out]
          n156 = call <vilib>:"Recursive File List.vi"("Folder Path"=w437) -> ("All Files in Dir"=w436:path[])  [unwired: 6 in, 4 out]
          n157 = for {
            tunnel: w436 -> [w447] mode=indexing
            shift-right: [w448] -> w433
            shift-left: refnum<vi>[] [] -> [w449]
            tunnel: w431 -> [w446]
            shift-right: [w444] -> w430
            shift-left: path[] [] -> [w445]
            tunnel: w428 -> [w442]
            n158 = Strip Path(path=w447) -> (name=w440:string)  [unwired: 1 out]
            n159 = for {
              tunnel: w440 -> [w453]
              tunnel: w446 -> [w452] mode=indexing
              tunnel: [w450] -> w443 mode=indexing
              n160 = Match Pattern(string=w453, regular expression=w452) -> (offset past match=w451:i32)  [unwired: 1 in, 3 out]
              n161 = Greater Or Equal To 0?(x=w451) -> (x >= 0?=w450:bool)
            }
            n162 = Match Pattern(string=w440, regular expression="GOOPKernel.vi") -> (offset past match=w438:i32)  [unwired: 1 in, 3 out]
            n163 = Or Array Elements(Boolean array=w443) -> (logical OR=w441:bool)
            n164 = case shown="False" w441 {
              tunnel: w447 -> [w454 w459]
              tunnel: w449 -> [w456 w463]
              tunnel: [w456 w462] -> w448
              tunnel: w445 -> [w455 w461]
              tunnel: [w455 w460] -> w444
              tunnel: w442 -> [_ w458]
              tunnel: w438 -> [_ w457]
              frame True {
                n165 = Delete(path (use dialog)=w454) -> ()  [unwired: 4 in, 3 out]
              }
              frame False {
                n166 = call <resource>:"Scripting_OpenViRef.vi"("ViPath/ViName/Viref"=w459, "AppRef"=w458) -> ("error out"=w465:errorcluster, "vi reference"=w464:refnum<vi>)  [unwired: 7 in, 1 out]
                n167 = case shown="No Error" w465 {
                  tunnel: w464 -> [w472 _]
                  tunnel: w463 -> [w471 w486]
                  tunnel: [w470 w486] -> w462
                  tunnel: w461 -> [w469 w485]
                  tunnel: [w468 w485] -> w460
                  tunnel: w459 -> [w467 _]
                  tunnel: w457 -> [w466 _]
                  frame No Error {
                    n168 = case shown="Default" w466 {
                      tunnel: w472 -> [w478 w484]
                      tunnel: w471 -> [w477 w483]
                      tunnel: [w476 w482] -> w470
                      tunnel: w469 -> [w475 w481]
                      tunnel: [w474 w480] -> w468
                      tunnel: w467 -> [w473 w479]
                      frame -1 {
                        n169 = Build Array (concatenate)(w475, w473) -> (w474:path[])
                        n170 = Build Array (concatenate)(w477, w478) -> (w476:refnum<vi>[])
                      }
                      frame Default {
                        n171 = Build Array (concatenate)(w479, w481) -> (w480:path[])
                        n172 = Build Array (concatenate)(w484, w483) -> (w482:refnum<vi>[])
                      }
                    }
                  }
                  frame Error {
                  }
                }
              }
            }
          }
          n173 = Bundle By Name(cluster=w434, "ViRefs"=w433, "ViPathes"=w430) -> (w432:T2)
        }
        n174 = property on="Progress" class="LstBox (strict)"() -> ("Item Names"=w419:string[])  [unwired: 2 in, 2 out]
        n175 = Build Array (concatenate)(w419, "Loading Class VIs in memory") -> (w418:string[])
        n176 = Bundle By Name(cluster=w426, "Classes"=w421) -> (w425:T7)
        n177 = property on="Progress" class="LstBox (strict)"("Item Names"=w418) -> ()  [unwired: 2 in, 2 out]
      }
      frame "AnalyseClass" {
        n178 = Unbundle By Name(w495) -> ("AppRef"=w493:refnum<vi>, "Classes"=w489:T2[])
        n179 = for {
          tunnel: w489 -> [w501] mode=indexing
          tunnel: [w498] -> w488 mode=indexing
          tunnel: [w497] -> w487 mode=indexing
          n180 = Unbundle By Name(w501) -> ("ClassFolder"=w498:path, "ClassName"=w499:string)
          n181 = Concatenate Strings(w499, ".lvclass" ("string")) -> (w497:string)
        }
        n182 = for {
          tunnel: w489 -> [w511] mode=indexing
          tunnel: [w510] -> w490 mode=indexing
          tunnel: w493 -> [w508]
          tunnel: w488 -> [w504]
          tunnel: w487 -> [w503]
          n183 = Unbundle By Name(w511) -> ("ClassFolder"=w516:path)
          n184 = call <vilib>:"Recursive File List.vi"("pattern"="*GoopKernel.vi", "Treat LLBs as Folders?"=TRUE, "Folder Path"=w516) -> ("All Files in Dir"=w514:path[])  [unwired: 4 in, 4 out]
          n185 = Index Array(array=w514) -> (element=w513:path)  [unwired: 1 in]
          n186 = call <resource>:"ConvertGoop2ToGoop3_GetGoop2ClassInheritance.vi"("application reference (local)"=w508, "Goop2VIPath(has to use GOOPKernel)"=w513) -> ("Inheritance"=w505:path[])  [unwired: 16 in, 1 out]
          n187 = Index Array(array=w505) -> (element=w509:path)  [unwired: 1 in]
          n188 = Delete From Array(array=w505) -> (deleted portion=w507:path)  [unwired: 2 in, 1 out]
          n189 = for {
            tunnel: w505 -> [w520] mode=indexing
            tunnel: w504 -> [w521]
            tunnel: w503 -> [w519]
            tunnel: [w517] -> w502 mode=indexing
            n190 = Search 1D Array(1D array=w521, element=w520) -> (index of element=w518:i32)  [unwired: 1 in]
            n191 = Index Array(array=w519, index=w518) -> (element=w517:string)
          }
          n192 = Array Size(array=w505) -> (size(s)=w506:i32)
          n193 = Bundle By Name(cluster=w511, "NoOfInheritance"=w506, "InheritsFrom"=w509, "RootClass"=w507, "AllInheritanceClasses"=w502) -> (w510:T2)
        }
        n194 = Sort 1D Array(array=w490) -> (sorted array=w491:T2[])
        n195 = Bundle By Name(cluster=w495, "Classes"=w491) -> (w494:T7)
      }
      frame "RemoveReentrantForDynamicDispatchVIs" {
        n196 = Unbundle By Name(w526) -> ("Classes"=w523:T2[])
        n197 = for {
          tunnel: w523 -> [w536] mode=indexing
          shift-right: [w534] -> w524
          shift-left: w525 -> [w535]
          tunnel: w523 -> [w531]
          i -> [w530]
          n198 = Delete From Array(array=w531, index=w530) -> (array with subset deleted=w529:T2[])  [unwired: 1 in, 1 out]
          n199 = Unbundle By Name(w536) -> ("ViRefs"=w533:refnum<vi>[], "ViPathes"=w532:path[])
          n200 = for {
            tunnel: w529 -> [w541] mode=indexing
            shift-right: [w539] -> w527
            shift-left: string[] [] -> [w540]
            n201 = Unbundle By Name(w541) -> ("ViPathes"=w537:path[])
            n202 = for {
              tunnel: [w543] -> w538 mode=indexing
              tunnel: w537 -> [w542] mode=indexing
              n203 = Strip Path(path=w542) -> (name=w543:string)  [unwired: 1 out]
            }
            n204 = Build Array (concatenate)(w540, w538) -> (w539:string[])
          }
          n205 = for {
            shift-right: [w556] -> w534
            shift-left: w535 -> [w557]
            tunnel: w533 -> [w555] mode=indexing
            tunnel: w532 -> [w554] mode=indexing
            tunnel: w527 -> [w547]
            n206 = Strip Path(path=w554) -> (stripped path=w553:path, name=w549:string)
            n207 = To Lower Case(string=w547) -> (all lower case string=w546:string[])
            n208 = To Lower Case(string=w549) -> (all lower case string=w548:string)
            n209 = Strip Path(path=w553) -> (name=w552:string)  [unwired: 1 out]
            n210 = Search 1D Array(1D array=w546, element=w548) -> (index of element=w545:i32)  [unwired: 1 in]
            n211 = Not Equal?(x=w552, y="utils") -> (x != y?=w550:bool)
            n212 = Greater Or Equal To 0?(x=w545) -> (x >= 0?=w544:bool)
            n213 = case shown="True" w550 {
              tunnel: w557 -> [w558 w559]
              tunnel: [w558 w559] -> w556
              tunnel: w555 -> [_ w561]
              tunnel: w544 -> [_ _]
              frame False {
              }
              frame True {
                n214 = property class="VI"(reference=w561, error in=w559, "Exec.IsReentrant"=FALSE ("Execution:Is Reentrant")) -> ()  [unwired: 2 out]
              }
            }
          }
        }
      }
      frame "RecompilingVIs" {
        n215 = call <resource>:"ConvertGoop2ToGoop3_RecompileAll.vi"("error IO 2"=w568, "Cluster 2"=w567) -> ("error IO"=w566:errorcluster)  [unwired: 7 in]
        n216 = property on="Progress" class="LstBox (strict)"() -> ("Item Names"=w564:string[])  [unwired: 2 in, 2 out]
        n217 = Build Array (concatenate)(w564, "Recompiling VIs") -> (w563:string[])
        n218 = property on="Progress" class="LstBox (strict)"("Item Names"=w563) -> ()  [unwired: 2 in, 2 out]
      }
      frame "AddVIsToProject" {
        n219 = Unbundle By Name(w571) -> ("ProjectRef"=w570:refnum<vi>, "My Computer"=w569:refnum<vi>)
        n220 = Unbundle By Name(w571) -> ("TopFolderPath"=w572:path, "VIsToRelink(Paths)"=w579:path[])
        n221 = for {
          tunnel: w579 -> [w581] mode=indexing
          shift-right: [w580] -> w574
          shift-left: w578 -> [w580]
          tunnel: w572 -> [w588]
          tunnel: w569 -> [w584]
          tunnel: w570 -> [w583]
          n222 = Strip Path(path=w581) -> (stripped path=w587:path, name=w582:string)
          n223 = call <vilib>:"Compare Two Paths.vi"("Path 2"=w587, "Path 1"=w588) -> ("Relative Path from 1 to 2"=w586:path)  [unwired: 6 in, 3 out]
          n224 = Path To String(path=w586) -> (string=w585:string)
          n225 = case shown="Default" w585 {
            selector: w585 -> [w602 _]
            tunnel: w584 -> [w601 w606]
            tunnel: w583 -> [w591 _]
            tunnel: w580 -> [w598 _]
            tunnel: w582 -> [w597 w607]
            tunnel: w581 -> [w596 w608]
            tunnel: [w592 w605] -> _
            frame Default {
              n226 = call <resource>:"GDSProject_CreateFolder.vi"("Project Refnum In"=w591, "Project Item To Create Folder Below(Use MyComputer if not wired)"=w601, "FolderName"=w602, "error in (no error)"=w598) -> ("ItemOut"=w590:refnum<vi>, "error out"=w599:errorcluster)  [unwired: 12 in, 2 out]
              n227 = invoke class="ProjectItem" method="AddItem"(reference=w590, error in=w599, "Name"=w597, "Path"=w596, "Type"="VI") -> (reference out=w594:refnum<vi>, error out=w595:errorcluster, "AddItem"=w589:refnum<vi>)  [unwired: 1 in, 3 out]
              n228 = Close Reference(reference=w594, error in (no error)=w595) -> (error out=w593:errorcluster)
              n229 = Close Reference(reference=w589, error in (no error)=w593) -> (error out=w592:errorcluster)
            }
            frame "", "." {
              n230 = invoke class="TargetItem" method="AddItem"(reference=w606, "Name"=w607, "Path"=w608, "Type"="VI") -> (error out=w603:errorcluster, "AddItem"=w604:refnum<vi>)  [unwired: 2 in, 4 out]
              n231 = Close Reference(reference=w604, error in (no error)=w603) -> (error out=w605:errorcluster)
            }
          }
        }
        n232 = property on="Progress" class="LstBox (strict)"() -> ("Item Names"=w577:string[])  [unwired: 2 in, 2 out]
        n233 = Build Array (concatenate)(w577, "Adding VIs to project") -> (w576:string[])
        n234 = property on="Progress" class="LstBox (strict)"("Item Names"=w576) -> ()  [unwired: 2 in, 2 out]
      }
      frame "RenameFiles" {
        n235 = Unbundle By Name(w611) -> ("My Computer"=w614:refnum<vi>, "TopFolderPath"=w619:path)
        n236 = Unbundle By Name(w611) -> ("Classes"=w620:T2[])
        n237 = for {
          tunnel: w620 -> [w643] mode=indexing
          tunnel: w619 -> [_]
          shift-right: [w629] -> w618
          shift-left: w617 -> [w622]
          tunnel: [w650] -> w615 mode=indexing
          tunnel: w614 -> [w628]
          shift-right: [w645] -> w613
          shift-left: path[] [] -> [w646]
          tunnel: w611 -> [w642]
          n238 = Unbundle By Name(w643) -> ("ClassName"=w625:string, "ClassFolder"=w647:path, "ClassPrefix"=w651:string, "ViRefs"=w644:refnum<vi>[])
          n239 = Unbundle By Name(w643) -> ("ClassName"=w648:string)
          n240 = Format Into String(format string="Renaming class: %s", w648) -> (resulting string=w633:string)  [unwired: 2 in, 1 out]
          n241 = property on="Progress" class="LstBox (strict)"() -> ("Item Names"=w641:string[], "Number of Rows"=w635:u32)  [unwired: 2 in, 2 out]
          n242 = Build Array (concatenate)(w641, w633) -> (w636:string[])
          n243 = Array Size(array=w636) -> (size(s)=w640:i32)
          n244 = Subtract(x=w640, y=w635) -> (x-y=w639:u32)
          n245 = To Long Integer(number=w639) -> (32bit integer=w637:i32)
          n246 = Max & Min(x=w637, y=0) -> (max(x,y)=w634:i32)  [unwired: 1 out]
          n247 = property on="Progress" class="LstBox (strict)"("Item Names"=w636, "Top Row"=w634) -> (error out=w632:errorcluster)  [unwired: 2 in, 1 out]
          n248 = for {
            tunnel: w644 -> [w677] mode=indexing
            shift-right: [w654] -> _
            shift-left: w622 -> [w654]
            tunnel: w651 -> [w675]
            tunnel: [w672] -> w630 mode=indexing
            tunnel: w647 -> [w671]
            tunnel: [w670] -> w624
            shift-right: [w668] -> w645
            shift-left: w646 -> [w667]
            tunnel: [w664] -> w626 mode=indexing
            tunnel: w642 -> [w661]
            tunnel: w632 -> [_]
            tunnel: [w655] -> _
            n249 = property class="VI"(reference=w677, error in=w654) -> (reference out=w676:refnum<vi>, error out=w663:errorcluster, "Path"=w669:path, "OwningApp"=w660:refnum<vi>)
            n250 = while {
              shift-right: [w678] -> w656
              shift-left: _ -> [w680]
              stop <- TRUE stop-if-true
              n251 = Increment(x=w680) -> (x+1=w679:i32)
              n252 = To Long Integer(number=w679) -> (32bit integer=w678:i32)
            }
            n253 = Strip Path(path=w669) -> ()  [unwired: 2 out]
            n254 = disable-structure shown="Disabled" {
              disable-tunnel: w663 -> [w685 w686]
              disable-tunnel: [w684 w686] -> w662
              disable-tunnel: w661 -> [w683 _]
              frame Disabled {
                n255 = call <resource>:"ConvertGoop2ToGoop3_RecompileAll.vi"("error IO 2"=w685, "Cluster 2"=w683) -> ("error IO"=w684:errorcluster)  [unwired: 7 in]
              }
              frame Enabled {
              }
            }
            n256 = property class="App"(reference=w660) -> (reference out=w653:refnum<vi>, error out=w652:errorcluster, "App.Name"=w659:string)  [unwired: 1 in]
            n257 = Format Into String(format string="TempName%d.", w656) -> (resulting string=w657:string)  [unwired: 2 in, 1 out]
            n258 = call <resource>:"ConvertGoop2ToGoop3_KeepViPrefix.vi"("OrgViName"=w669, "ClassFolder"=w671, "error in (no error)"=w662, "ClassPrefix"=w675) -> ("ClassFolderOut"=w670:path, "Don'tUseVI"=w665:bool, "NewClassPath"=w666:path, "NewClassPathWithPreFix"=w674:path, "error out"=w673:errorcluster)  [unwired: 10 in, 1 out]
            n259 = Close Reference(reference=w653, error in (no error)=w652) -> ()  [unwired: 1 out]
            n260 = case shown="False" w665 {
              tunnel: w676 -> [w706 w742]
              tunnel: w674 -> [w695 _]
              tunnel: w673 -> [w704 w739]
              tunnel: [w701 w737] -> w655
              tunnel: w666 -> [w692 _]
              tunnel: [w703 w738] -> w672
              tunnel: w669 -> [w700 w738]
              tunnel: w669 -> [_ w734]
              tunnel: [w699 w735] -> w668
              tunnel: w667 -> [w698 w736]
              tunnel: [w697 _] -> w664
              tunnel: w659 -> [w693 _]
              tunnel: w657 -> [w690 _]
              frame False {
                # "Remove\nPrefix ?"
                n261 = call <vilib>:"Get File Extension.vi"("file"=w692) -> ("filename without extension"=w691:string, "lowercase file extension"=w689:string)  [unwired: 7 in, 2 out]
                n262 = Strip Path(path=w695) -> (name=w694:string)  [unwired: 1 out]
                n263 = invoke class="VI" method="Save.Instrument"(reference=w706, error in=w704, "Path to saved file"=w692) -> (reference out=w697:refnum<vi>, error out=w705:errorcluster)  [unwired: 3 in, 4 out]
                n264 = Strip Path(path=w692) -> (stripped path=w688:path, name=w696:string)
                n265 = Concatenate Strings(w691, w690, w689) -> (w687:string)
                n266 = case shown="Error" w705 {
                  selector: w705 -> [w712 _]
                  tunnel: [w712 w719] -> w701
                  tunnel: w695 -> [_ w720]
                  tunnel: w704 -> [_ w722]
                  tunnel: w697 -> [_ w721]
                  tunnel: [w711 w720] -> w703
                  tunnel: w692 -> [w711 _]
                  tunnel: w696 -> [_ w718]
                  tunnel: w694 -> [_ w717]
                  tunnel: w693 -> [_ w716]
                  tunnel: w688 -> [_ w715]
                  tunnel: w687 -> [_ w714]
                  frame No Error {
                    # "Prefix\nRemoved"
                  }
                  frame Error {
                    # "..not\npossible"
                    n267 = Build Path(base path=w715, name or relative path=w714) -> (appended path=w713:path)
                    n268 = stacked-sequence {
                      tunnel: w718 -> [w725]
                      tunnel: w717 -> [w724]
                      tunnel: [w724] -> _
                      tunnel: w716 -> [w723]
                      frame #0 {
                        w729 = path "c:/G2To3.txt" ("file (use dialog)")
                        n269 = Read from Text File(file (use dialog)=w729) -> (text=w726:string)  [unwired: 3 in, 3 out]
                        n270 = Format Into String(format string="       %s(%s)%s\n", initial string=w726, w725, w724, w723) -> (resulting string=w728:string)  [unwired: 1 in, 1 out]
                        n271 = stacked-sequence {
                          tunnel: w728 -> [w732]
                          tunnel: w729 -> [w730]
                          frame #0 {
                            n272 = Delete(path (use dialog)=w730) -> (deleted path=w731:path)  [unwired: 4 in, 2 out]
                            n273 = Write to Text File(file (use dialog)=w731, text=w732) -> ()  [unwired: 2 in, 3 out]
                          }
                        }
                      }
                    }
                    n274 = invoke class="VI" method="Save.Instrument"(reference=w721, error in=w722, "Path to saved file"=w713) -> (error out=w719:errorcluster)  [unwired: 3 in, 5 out]
                  }
                }
                n275 = Not Equal?(x=w703, y=w700) -> (x != y?=w702:bool)
                n276 = case shown="False" w702 {
                  tunnel: w701 -> [_ _]
                  tunnel: w700 -> [_ w708]
                  tunnel: [w707 w710] -> w699
                  tunnel: w698 -> [w707 w709]
                  frame False {
                  }
                  frame True {
                    n277 = Build Array (concatenate)(w709, w708) -> (w710:path[])
                  }
                }
              }
              frame True {
                n278 = case shown="False" FALSE {
                  tunnel: w742 -> [w744 w748]
                  tunnel: [w744 w747] -> w741
                  tunnel: [w743 w746] -> w740
                  tunnel: w739 -> [w743 w745]
                  frame False {
                  }
                  frame True {
                    n279 = invoke class="VI" method="Save.Instrument"(reference=w748, error in=w745) -> (reference out=w747:refnum<vi>, error out=w746:errorcluster)  [unwired: 4 in, 4 out]
                  }
                }
                n280 = Close Reference(reference=w741, error in (no error)=w740) -> (error out=w737:errorcluster)
                n281 = Build Array (concatenate)(w736, w734) -> (w735:path[])
              }
            }
            n282 = stacked-sequence {
              tunnel: w655 -> [_]
              frame #0 {
                n283 = Wait (ms)(milliseconds to wait=u32 2) -> ()  [unwired: 1 out]
              }
            }
          }
          n284 = call <resource>:"ConvertGoop2ToGoop3_CreateLvClass.vi"("ClassFolder"=w624, "ProjectItem"=w628, "ClassName"=w625, "ViRefsIn"=w626, "ViPathsIn"=w630, "error in"=w622) -> ("LvClassCreated"=w623:refnum<vi>, "ViRefsOut"=w627:refnum<vi>[], "ViPathsOut"=w631:path[], "error out"=w629:errorcluster)  [unwired: 6 in]
          n285 = Bundle By Name(cluster=w643, "ClassFolder"=w624, "ViRefs"=w627, "ViPathes"=w631, "ClassRef"=w623) -> (w650:T2)
        }
        n286 = Bundle By Name(cluster=w611, "Classes"=w615) -> (w616:T7)
        n287 = for {
          tunnel: w613 -> [w621] mode=indexing
          n288 = Delete(path (use dialog)=w621) -> ()  [unwired: 4 in, 3 out]
        }
      }
      frame "RenameTempNames" {
        n289 = Unbundle By Name(w750) -> ("Classes"=w753:T2[])
        n290 = for {
          tunnel: w753 -> [w755] mode=indexing
          shift-right: [w754] -> w752
          shift-left: w749 -> [w758]
          tunnel: w750 -> [w756]
          n291 = Unbundle By Name(w755) -> ("ViRefs"=w757:refnum<vi>[])
          n292 = for {
            tunnel: w757 -> [w764] mode=indexing
            shift-right: [w761] -> w754
            shift-left: w758 -> [w759]
            tunnel: w756 -> [_]
            n293 = property class="VI"(reference=w764, error in=w759) -> (reference out=w762:refnum<vi>, error out=w760:errorcluster, "Path"=w763:path)
            n294 = case shown="No Error" w760 {
              selector: w760 -> [w765 _]
              tunnel: w763 -> [w769 _]
              tunnel: w762 -> [w768 _]
              tunnel: [w767 w784] -> w761
              tunnel: w759 -> [_ w784]
              frame No Error {
                n295 = call <vilib>:"Get File Extension.vi"("file"=w769) -> ("filename without extension"=w773:string)  [unwired: 7 in, 3 out]
                n296 = Match Pattern(string=w773, regular expression="TempName[0-9]+") -> (before substring=w771:string, after substring=w770:string, offset past match=w766:i32)  [unwired: 1 in, 1 out]
                n297 = case shown="0, Default" w766 {
                  tunnel: w771 -> [w782 _]
                  tunnel: w770 -> [w781 _]
                  tunnel: w769 -> [w780 _]
                  tunnel: w768 -> [w777 _]
                  tunnel: w765 -> [w776 w783]
                  tunnel: [w775 w783] -> w767
                  frame 0, Default {
                    n298 = Concatenate Strings(w782, w781) -> (w778:string)
                    n299 = Strip Path(path=w780) -> (stripped path=w779:path)  [unwired: 1 out]
                    n300 = Build Path(base path=w779, name or relative path=w778) -> (appended path=w774:path)
                    n301 = invoke class="VI" method="Save.Instrument"(reference=w777, error in=w776, "Path to saved file"=w774) -> (error out=w775:errorcluster)  [unwired: 3 in, 5 out]
                  }
                  frame -1 {
                  }
                }
              }
              frame Error {
              }
            }
          }
        }
      }
      frame "FindAllCallParentMethodCalls" {
        n302 = Unbundle By Name(w789) -> ("Classes"=w792:T2[])
        n303 = for {
          tunnel: w792 -> [w799] mode=indexing
          shift-right: [w797] -> w790
          shift-left: w791 -> [w810]
          shift-right: [w793] -> w787
          shift-left: cluster{"VI Refnum":refnum<vi>, "Position":T6}[] [] -> [w794]
          n304 = Unbundle By Name(w799) -> ("ClassName"=w798:string)
          n305 = Unbundle By Name(w799) -> ("ViRefs"=w796:refnum<vi>[], "AllInheritanceClasses"=w795:string[])
          n306 = for {
            shift-right: [w816] -> w797
            shift-left: w810 -> [w818]
            tunnel: w795 -> [w817]
            tunnel: w796 -> [w813] mode=indexing
            shift-right: [w814] -> w793
            shift-left: w794 -> [w815]
            # "Does this VI call a Parent Method VI with te same name,\nIf so It shoule be peplaced by a CallParentMethod-function"
            n307 = Not A Number/Path/Refnum?(number/path/refnum=w813) -> (NaN/Path/Refnum?=w812:bool)
            n308 = case shown="False" w812 {
              tunnel: w818 -> [w834 w872]
              tunnel: w817 -> [w833 _]
              tunnel: [w824 w872] -> w816
              tunnel: w815 -> [w822 w871]
              tunnel: [w821 w871] -> w814
              tunnel: w813 -> [w820 _]
              frame False {
                n309 = property class="VI"(reference=w820, error in=w834) -> (reference out=w823:refnum<vi>, error out=w825:errorcluster, "VIType"=w826:T13, "Callees"=w831:string[], "Name"=w829:string)
                n310 = Match Pattern(string=w829, regular expression=":") -> (after substring=w827:string)  [unwired: 1 in, 3 out]
                n311 = for {
                  tunnel: w833 -> [w870] mode=indexing
                  tunnel: w827 -> [w869]
                  tunnel: [w867] -> w819 mode=indexing
                  n312 = Concatenate Strings(w870, ":" ("string"), w869) -> (w867:string)
                }
                n313 = To Lower Case(string=w831) -> (all lower case string=w830:string[])
                n314 = To Lower Case(string=w819) -> (all lower case string=w832:string[])
                n315 = case shown="\"Standard VI\"" w826 {
                  tunnel: w832 -> [_ w846]
                  tunnel: w830 -> [_ w845]
                  tunnel: w825 -> [w836 w842]
                  tunnel: [w836 w841] -> w824
                  tunnel: w819 -> [_ w837]
                  tunnel: w823 -> [_ w840]
                  tunnel: w822 -> [w835 w839]
                  tunnel: [w835 w838] -> w821
                  frame Default {
                  }
                  frame "Standard VI" {
                    n316 = for {
                      tunnel: w846 -> [w865] mode=indexing
                      tunnel: w845 -> [w866]
                      tunnel: [w863] -> w844 mode=indexing
                      n317 = Search 1D Array(1D array=w866, element=w865) -> (index of element=w864:i32)  [unwired: 1 in]
                      n318 = Greater Or Equal To 0?(x=w864) -> (x >= 0?=w863:bool)
                    }
                    n319 = Or Array Elements(Boolean array=w844) -> (logical OR=w843:bool)
                    n320 = case shown="True" w843 {
                      tunnel: w842 -> [w847 w855]
                      tunnel: [w847 w854] -> w841
                      tunnel: w837 -> [_ w853]
                      tunnel: w840 -> [_ w850]
                      tunnel: w839 -> [w848 w851]
                      tunnel: [w848 w849] -> w838
                      frame False {
                      }
                      frame True {
                        n321 = call <resource>:"Scripting_FindVisOnDiagram.vi"("ViRef"=w850, "VIsToSerachFor/ViName"=w853, "error in (no error)"=w855) -> ("VisFound"=w852:refnum<vi>[], "error out"=w854:errorcluster)  [unwired: 15 in]
                        n322 = for {
                          tunnel: w852 -> [w862] mode=indexing
                          shift-right: [w857] -> w849
                          shift-left: w851 -> [w859]
                          tunnel: w850 -> [w860]
                          n323 = property class="GObj"(reference=w862) -> (reference out=w856:refnum<vi>, "Position"=w861:T6)  [unwired: 1 in, 1 out]
                          n324 = Bundle("VI Refnum"=w860, "Position"=w861) -> (w858:cluster{"VI Refnum":refnum<vi>, "Position":T6})  [unwired: 1 in]
                          n325 = Build Array (concatenate)(w859, w858) -> (w857:cluster{"VI Refnum":refnum<vi>, "Position":T6}[])
                          n326 = Close Reference(reference=w856) -> ()  [unwired: 1 in, 1 out]
                        }
                      }
                    }
                  }
                }
              }
              frame True {
              }
            }
          }
          n327 = Format Into String(format string="Searching Call Parent Method: %s", w798) -> (resulting string=w801:string)  [unwired: 2 in, 1 out]
          n328 = property on="Progress" class="LstBox (strict)"() -> ("Item Names"=w809:string[], "Number of Rows"=w803:u32)  [unwired: 2 in, 2 out]
          n329 = Build Array (concatenate)(w809, w801) -> (w804:string[])
          n330 = Array Size(array=w804) -> (size(s)=w808:i32)
          n331 = Subtract(x=w808, y=w803) -> (x-y=w807:u32)
          n332 = To Long Integer(number=w807) -> (32bit integer=w805:i32)
          n333 = Max & Min(x=w805, y=0) -> (max(x,y)=w802:i32)  [unwired: 1 out]
          n334 = property on="Progress" class="LstBox (strict)"("Item Names"=w804, "Top Row"=w802) -> ()  [unwired: 2 in, 2 out]
          n335 = stacked-sequence {
            tunnel: w797 -> [_]
            frame #0 {
              n336 = Wait (ms)(milliseconds to wait=u32 5) -> ()  [unwired: 1 out]
            }
          }
        }
        n337 = Bundle By Name(cluster=w789, "CallParentMethod"=w787) -> (w788:T7)
      }
      frame "UpdateNewVI" {
        n338 = Unbundle By Name(w873) -> ("Classes"=w887:T2[])
        n339 = call <resource>:"ConvertGoop2ToGoop3_RecompileAll.vi"("error IO 2"=w875, "Cluster 2"=w873) -> ("error IO"=w874:errorcluster)  [unwired: 7 in]
        n340 = for {
          tunnel: w887 -> [w898] mode=indexing
          shift-right: [w896] -> w886
          shift-left: w874 -> [w897]
          n341 = Unbundle By Name(w898) -> ("ViRefs"=w895:refnum<vi>[], "ClassFolder"=w894:path, "ClassName"=w893:string)
          n342 = Concatenate Strings(w893, "_New.vi" ("string")) -> (w889:string)
          n343 = Build Path(base path=w894, name or relative path="Utils") -> (appended path=w891:path)
          n344 = Build Path(base path=w891, name or relative path=w889) -> (appended path=w888:path)
          n345 = for {
            tunnel: w895 -> [w904] mode=indexing
            shift-right: [w899] -> w896
            shift-left: w897 -> [w909]
            tunnel: w888 -> [w905]
            n346 = property class="VI"(reference=w904) -> ("Name"=w903:string)  [unwired: 1 in, 2 out]
            n347 = Match Pattern(string=w903, regular expression="_Create\\2Evi$") -> (offset past match=w901:i32)  [unwired: 1 in, 3 out]
            n348 = call <resource>:"Scripting_ConnecorPaneRewiring.vi"("ViRef"=w904, "SubViThatHasChangedConnectorPane"=w905, "OldConnectorPaneIndex"=u32[] [6], "NewConnectorPaneIndex"=u32[] [8], "error in (no error)"=w909) -> ("error out"=w906:errorcluster)  [unwired: 14 in]
            n349 = case shown="-1" w901 {
              tunnel: w906 -> [w910 w915]
              tunnel: [w910 w914] -> w900
              tunnel: w905 -> [_ w912]
              tunnel: w904 -> [_ w911]
              frame 0, Default {
              }
              frame -1 {
                n350 = call <resource>:"Scripting_ConnecorPaneCreateConstant.vi"("ViRef"=w911, "SubViThatHasChangedConnectorPane"=w912, "ConnectorPaneIndexToCReateConstantsOn"=u32[] [6, 0] ("OldConnectorPaneIndex"), "error in (no error)"=w915) -> ("error out"=w914:errorcluster)  [unwired: 15 in]
              }
            }
            n351 = call <vilib>:"Clear Errors.vi"("error in (no error)"=w900) -> ("error out"=w899:errorcluster)  [unwired: 5 in, 1 out]
            n352 = stacked-sequence {
              tunnel: w899 -> [_]
              frame #0 {
                n353 = Wait (ms)(milliseconds to wait=u32 2) -> ()  [unwired: 1 out]
              }
            }
          }
        }
        n354 = property on="Progress" class="LstBox (strict)"() -> ("Item Names"=w884:string[], "Number of Rows"=w878:u32)  [unwired: 2 in, 2 out]
        n355 = Build Array (concatenate)(w884, "Update NEW-VI (due to cone-pane changes)") -> (w879:string[])
        n356 = Array Size(array=w879) -> (size(s)=w883:i32)
        n357 = Subtract(x=w883, y=w878) -> (x-y=w882:u32)
        n358 = To Long Integer(number=w882) -> (32bit integer=w880:i32)
        n359 = Max & Min(x=w880, y=0) -> (max(x,y)=w877:i32)  [unwired: 1 out]
        n360 = property on="Progress" class="LstBox (strict)"("Item Names"=w879, "Top Row"=w877) -> ()  [unwired: 2 in, 2 out]
      }
      frame "SetInheritance" {
        n361 = Unbundle By Name(w922) -> ("Classes"=w920:T2[])
        n362 = for {
          tunnel: w920 -> [w926] mode=indexing
          tunnel: [w925] -> w919 mode=indexing
          tunnel: [w924] -> w918 mode=indexing
          n363 = Unbundle By Name(w926) -> ("ClassName"=w925:string, "ClassRef"=w924:refnum<vi>)
        }
        n364 = for {
          tunnel: w920 -> [w942] mode=indexing
          shift-right: [w927] -> w923
          shift-left: w921 -> [w937]
          tunnel: w919 -> [w939]
          tunnel: w918 -> [w938]
          n365 = Unbundle By Name(w942) -> ("ClassName"=w932:string, "ClassRef"=w941:refnum<vi>, "InheritsFrom"=w940:path)
          n366 = Strip Path(path=w940) -> (name=w935:string)  [unwired: 1 out]
          n367 = Match Pattern(string=w935, regular expression="_[Cc][Ll][Aa][Ss][Ss]") -> (before substring=w930:string)  [unwired: 1 in, 3 out]
          n368 = Match Pattern(string=w930, regular expression="[.][Ll][Ll][Bb]$") -> (before substring=w928:string)  [unwired: 1 in, 3 out]
          n369 = Format Into String(format string="Setting inheritance: %s->%s", w932, w928) -> (resulting string=w931:string)  [unwired: 2 in, 1 out]
          n370 = Search 1D Array(1D array=w939, element=w928) -> (index of element=w936:i32)  [unwired: 1 in]
          n371 = case shown="0, Default" w936 {
            tunnel: w941 -> [w960 _]
            tunnel: w936 -> [w959 _]
            tunnel: w938 -> [w958 _]
            tunnel: w937 -> [w956 w961]
            tunnel: [w953 w961] -> w927
            tunnel: w931 -> [w944 _]
            frame 0, Default {
              n372 = Index Array(array=w958, index=w959) -> (element=w957:refnum<vi>)
              n373 = property class="LVClassLibrary"(reference=w960, error in=w956, "Parent"=w957) -> (reference out=w955:refnum<vi>, error out=w954:errorcluster)
              n374 = property on="Progress" class="LstBox (strict)"() -> ("Item Names"=w952:string[], "Number of Rows"=w946:u32)  [unwired: 2 in, 2 out]
              n375 = Build Array (concatenate)(w952, w944) -> (w947:string[])
              n376 = Array Size(array=w947) -> (size(s)=w951:i32)
              n377 = Subtract(x=w951, y=w946) -> (x-y=w950:u32)
              n378 = To Long Integer(number=w950) -> (32bit integer=w948:i32)
              n379 = Max & Min(x=w948, y=0) -> (max(x,y)=w945:i32)  [unwired: 1 out]
              n380 = invoke class="LVClassLibrary" method="Save"(reference=w955, error in=w954) -> (error out=w953:errorcluster)  [unwired: 2 in, 3 out]
              n381 = property on="Progress" class="LstBox (strict)"("Item Names"=w947, "Top Row"=w945) -> ()  [unwired: 2 in, 2 out]
            }
            frame -1 {
            }
          }
          n382 = stacked-sequence {
            tunnel: w927 -> [_]
            frame #0 {
              n383 = Wait (ms)(milliseconds to wait=u32 2) -> ()  [unwired: 1 out]
            }
          }
        }
      }
      frame "UpdateLvClassIcon" {
        n384 = Unbundle By Name(w976) -> ("Classes"=w975:T2[], "AppRef"=w971:refnum<vi>)
        n385 = for {
          tunnel: w975 -> [w1019] mode=indexing
          shift-right: [w978] -> w974
          shift-left: w973 -> [w993]
          tunnel: w971 -> [w985]
          n386 = Unbundle By Name(w1019) -> ("ClassRef"=w986:refnum<vi>, "ClassFolder"=w1008:path)
          n387 = List Folder(path=w1008, pattern="*.vi") -> (filenames=w1010:string[])  [unwired: 2 in, 3 out]
          n388 = Index Array(array=w1010) -> (element=w1009:string)  [unwired: 1 in]
          n389 = Build Path(base path=w1008, name or relative path=w1009) -> (appended path=w992:path)
          n390 = call <resource>:"Scripting_OpenViRef.vi"("error in"=w993, "ViPath/ViName/Viref"=w992, "AppRef"=w985) -> ("error out"=w994:errorcluster, "vi reference"=w990:refnum<vi>)  [unwired: 6 in, 1 out]
          n391 = call <resource>:"GDSLvIcon_AnalyseViIcon.vi"("ViRef/LvCLassRef/LvLibRef/ViPath"=w990, "error in (no error)"=w994) -> ("FrameColor"=w1007:u32, "FrameThickness(1)"=w1005:u32, "HeaderIcon"=w1000:u8[][], "HeaderBkColor"=w995:u32, "BodyBkColor"=w1006:u32, "error out"=w991:errorcluster)  [unwired: 5 in, 7 out]
          n392 = Array Size(array=w1000) -> (size(s)=w999:i32[])
          n393 = Close Reference(reference=w990, error in (no error)=w991) -> ()  [unwired: 1 out]
          n394 = Index Array(array=w999) -> (element=w997:i32)  [unwired: 1 in]
          n395 = Subtract(x=u32 32 ("Width(30)"), y=w997) -> (x-y=w996:u32)
          n396 = Multiply(x=w1005, y=u32 2) -> (x*y=w1003:u32)
          n397 = Subtract(x=u32 32 ("Width(30)"), y=w1003) -> (x-y=w1001:u32)
          n398 = call <resource>:"GDSLvIcon_GenerateObjectIcon.vi"("HeaderColor"=w995, "BackgroundColor"=w1006, "Height"=w996, "error in (no error)"=w991, "Type"=enum16{"LvClass", "Library", "X-Control"}."LvClass", "Width(30)"=w1001) -> ("BodyIconOut"=w1012:u8[][], "error out"=w1013:errorcluster)  [unwired: 12 in]
          n399 = call <resource>:"GDSLvIcon_CreateIconPicture.vi"("FrameColor"=w1007, "FrameThickness(1)"=w1005, "HeaderIconIn"=w1000, "BodyIconIn"=w1012, "error in (no error)"=w1013) -> ("WholeIconOut"=w1017:u8[][], "error out"=w1014:errorcluster)  [unwired: 9 in, 4 out]
          n400 = Reshape Array(w1017, 1024 ("dimension size")) -> (w1015:u8[])
          n401 = Bundle By Name(cluster=T9 {"image type"=0, "image depth"=8, "image"=[], "mask"=[], "colors"=[], "Rectangle"={"left"=0, "top"=0, "right"=32, "bottom"=32}} ("image data"), "image"=w1015) -> (w988:T9)
          n402 = invoke class="LVClassLibrary" method="Set Icon"(reference=w986, error in=w1014, "color"=w988) -> (reference out=w981:refnum<vi>, error out=w982:errorcluster)  [unwired: 2 in, 3 out]
          n403 = property class="LVClassLibrary"(reference=w981, error in=w982) -> (reference out=w980:refnum<vi>, error out=w987:errorcluster, "Member Data"=w989:refnum<vi>)
          n404 = invoke class="VI" method="VI Icon.Set from Image Data"(reference=w989, error in=w987, "ImageData"=w988) -> (reference out=w983:refnum<vi>, error out=w984:errorcluster)  [unwired: 3 in, 4 out]
          n405 = Close Reference(reference=w983, error in (no error)=w984) -> (error out=w979:errorcluster)
          n406 = invoke class="LVClassLibrary" method="Save"(reference=w980, error in=w979) -> (error out=w978:errorcluster)  [unwired: 2 in, 3 out]
          n407 = stacked-sequence {
            tunnel: w978 -> [_]
            frame #0 {
              n408 = Wait (ms)(milliseconds to wait=u32 2) -> ()  [unwired: 1 out]
            }
          }
        }
        n409 = property on="Progress" class="LstBox (strict)"() -> ("Item Names"=w970:string[], "Number of Rows"=w964:u32)  [unwired: 2 in, 2 out]
        n410 = Build Array (concatenate)(w970, string[] ["Updating Icons"] ("element")) -> (w965:string[])
        n411 = Array Size(array=w965) -> (size(s)=w969:i32)
        n412 = Subtract(x=w969, y=w964) -> (x-y=w968:u32)
        n413 = To Long Integer(number=w968) -> (32bit integer=w966:i32)
        n414 = Max & Min(x=w966, y=0) -> (max(x,y)=w963:i32)  [unwired: 1 out]
        n415 = property on="Progress" class="LstBox (strict)"("Item Names"=w965, "Top Row"=w963) -> ()  [unwired: 2 in, 2 out]
      }
      frame "UpdateLvClassAttributes" {
        n416 = Unbundle By Name(w1023) -> ("Classes"=w1025:T2[])
        n417 = for {
          tunnel: w1025 -> [w1042] mode=indexing
          shift-right: [w1040] -> w1024
          shift-left: w1022 -> [w1040]
          n418 = Unbundle By Name(w1042) -> ("ClassName"=w1027:string, "ClassRef"=w1041:refnum<vi>)
          n419 = call <resource>:"Scripting_PlaceGoopRefInClassAttribute.vi"("error in"=w1040, "ClassRefnum"=w1041) -> ("error out"=w1039:errorcluster, "ClusterTypeDefPath"=w1037:path, "ObjectRef.ctl"=w1038:path)  [unwired: 2 in, 1 out]
          n420 = case shown="Error" w1039 {
            tunnel: w1027 -> [_ w1048]
            tunnel: w1038 -> [_ w1046]
            tunnel: w1037 -> [_ w1044]
            frame No Error {
              n421 = stacked-sequence {
                frame #0 {
                  n422 = Wait (ms)(milliseconds to wait=u32 2) -> ()  [unwired: 1 out]
                }
              }
            }
            frame Error {
              w1052 = path "c:/G2To3.txt" ("file (use dialog)")
              n423 = Path To String(path=w1044) -> (string=w1045:string)
              n424 = Path To String(path=w1046) -> (string=w1047:string)
              n425 = Read from Text File(file (use dialog)=w1052) -> (text=w1049:string)  [unwired: 3 in, 3 out]
              n426 = Format Into String(format string="       Error %s(%s)%s\n", initial string=w1049, w1048, w1045, w1047) -> (resulting string=w1051:string)  [unwired: 1 in, 1 out]
              n427 = stacked-sequence {
                tunnel: w1051 -> [w1055]
                tunnel: w1052 -> [w1053]
                frame #0 {
                  n428 = Delete(path (use dialog)=w1053) -> (deleted path=w1054:path)  [unwired: 4 in, 2 out]
                  n429 = Write to Text File(file (use dialog)=w1054, text=w1055) -> ()  [unwired: 2 in, 3 out]
                }
              }
              n430 = call <vilib>:"Beep.vi"() -> ()  [unwired: 12 in]
            }
          }
          n431 = Format Into String(format string="Updating LvClass Attribute: %s", w1027) -> (resulting string=w1026:string)  [unwired: 2 in, 1 out]
          n432 = property on="Progress" class="LstBox (strict)"() -> ("Item Names"=w1036:string[], "Number of Rows"=w1030:u32)  [unwired: 2 in, 2 out]
          n433 = Build Array (concatenate)(w1036, w1026) -> (w1031:string[])
          n434 = Array Size(array=w1031) -> (size(s)=w1035:i32)
          n435 = Subtract(x=w1035, y=w1030) -> (x-y=w1034:u32)
          n436 = To Long Integer(number=w1034) -> (32bit integer=w1032:i32)
          n437 = Max & Min(x=w1032, y=0) -> (max(x,y)=w1029:i32)  [unwired: 1 out]
          n438 = property on="Progress" class="LstBox (strict)"("Item Names"=w1031, "Top Row"=w1029) -> ()  [unwired: 2 in, 2 out]
        }
      }
      frame "UpdateUtilsVIs" {
        n439 = Unbundle By Name(w1056) -> ("Classes"=w1064:T2[])
        n440 = local read "State"() -> (w1061:string)
        n441 = for {
          tunnel: w1064 -> [w1067] mode=indexing
          shift-right: [w1085] -> w1058
          shift-left: w1063 -> [w1086]
          tunnel: w1061 -> [w1069]
          tunnel: [w1065] -> w1060 mode=indexing
          n442 = Unbundle By Name(w1067) -> ("InheritsFrom"=w1093:path, "ClassName"=w1079:string, "ViRefs"=w1084:refnum<vi>[], "ViPathes"=w1082:path[])
          n443 = Empty String/Path?(string/path=w1093) -> (empty?=w1092:bool)
          n444 = Select(t=EndevoTemplateNames."BaseTemplate" ("TemplateNames"), s=w1092, f=EndevoTemplateNames."SubTemplate" ("TemplateNames")) -> (s? t:f=w1089:T10)
          n445 = Format Into String(w1089) -> (resulting string=w1081:string)  [unwired: 3 in, 1 out]
          n446 = call <resource>:"GOOP300_GetClassTemplatePath.vi"("ClassTemplateSubDirectory"=w1081) -> ("FolderPathOut"=w1087:path)  [unwired: 17 in, 1 out]
          n447 = Build Path(base path=w1087, name or relative path="utils") -> (appended path=w1083:path)
          n448 = for {
            shift-right: [w1105] -> w1085
            shift-left: w1086 -> [w1106]
            tunnel: w1084 -> [w1104] mode=indexing
            tunnel: w1083 -> [w1103]
            tunnel: w1082 -> [w1102] mode=indexing
            tunnel: w1081 -> [w1100]
            shift-right: [w1096] -> _
            shift-left: w1069 -> [w1097]
            shift-right: [w1095] -> w1066
            shift-left: "1.0.0" ("TemplateVersionUsed") -> [w1094]
            n449 = Strip Path(path=w1102) -> (stripped path=w1099:path, name=w1101:string)
            n450 = Strip Path(path=w1099) -> (name=w1098:string)  [unwired: 1 out]
            n451 = case shown="\"utils\"" w1098 {
              tunnel: w1106 -> [w1109 w1127]
              tunnel: [w1109 w1126] -> w1105
              tunnel: w1104 -> [_ w1125]
              tunnel: w1103 -> [_ w1124]
              tunnel: w1101 -> [_ w1115]
              tunnel: w1100 -> [_ w1122]
              tunnel: w1097 -> [w1108 w1118]
              tunnel: [w1108 w1116] -> w1096
              tunnel: [w1107 w1111] -> w1095
              tunnel: w1094 -> [w1107 w1110]
              frame Default {
              }
              frame "utils" {
                w1123 = "_" ("regular expression")
                n452 = Reverse String(1:w1115) -> (0:w1114:string)
                n453 = Match Pattern(string=w1114, regular expression=w1123) -> (before substring=w1113:string)  [unwired: 1 in, 3 out]
                n454 = Concatenate Strings(w1118, "." ("string")) -> (w1116:string)
                n455 = Reverse String(1:w1113) -> (0:w1112:string)
                n456 = local write "State"(w1116) -> ()
                n457 = Concatenate Strings(w1122, w1123, w1112) -> (w1121:string)
                n458 = Build Path(base path=w1124, name or relative path=w1121) -> (appended path=w1120:path)
                n459 = File/Directory Info(path=w1120) -> (size=w1119:i64)  [unwired: 1 in, 6 out]
                n460 = case shown="1.." w1119 {
                  tunnel: w1127 -> [w1129 w1132]
                  tunnel: [w1129 w1132] -> w1126
                  tunnel: w1125 -> [_ w1134]
                  tunnel: w1120 -> [_ w1133]
                  tunnel: [w1128 w1130] -> w1111
                  tunnel: w1110 -> [w1128 _]
                  frame 0, Default {
                  }
                  frame 1.. {
                    n461 = call <resource>:"Scripting_UpdateViFromTemplate.vi"("ViRef"=w1134, "TemplateVI(Path or Ref)"=w1133, "error in (no error)"=w1132) -> ("TemplateVersionUsed"=w1130:string, "error out"=w1131:errorcluster)  [unwired: 15 in]
                    n462 = stacked-sequence {
                      tunnel: w1131 -> [_]
                      frame #0 {
                        n463 = Wait (ms)(milliseconds to wait=u32 5) -> ()  [unwired: 1 out]
                      }
                    }
                  }
                }
              }
            }
          }
          n464 = Format Into String(format string="Updating utils VIs: %s", w1079) -> (resulting string=w1070:string)  [unwired: 2 in, 1 out]
          n465 = property on="Progress" class="LstBox (strict)"() -> ("Item Names"=w1078:string[], "Number of Rows"=w1072:u32)  [unwired: 2 in, 2 out]
          n466 = Build Array (concatenate)(w1078, w1070) -> (w1073:string[])
          n467 = Array Size(array=w1073) -> (size(s)=w1077:i32)
          n468 = Subtract(x=w1077, y=w1072) -> (x-y=w1076:u32)
          n469 = To Long Integer(number=w1076) -> (32bit integer=w1074:i32)
          n470 = Max & Min(x=w1074, y=0) -> (max(x,y)=w1071:i32)  [unwired: 1 out]
          n471 = property on="Progress" class="LstBox (strict)"("Item Names"=w1073, "Top Row"=w1071) -> ()  [unwired: 2 in, 2 out]
          n472 = Bundle By Name(cluster=w1067, "TemplateVersionUsed"=w1066) -> (w1065:T2)
        }
        n473 = Bundle By Name(cluster=w1056, "Classes"=w1060) -> (w1059:T7)
        n474 = call <resource>:"ConvertGoop2ToGoop3_RecompileAll.vi"("error IO 2"=w1058, "Cluster 2"=w1056) -> ("error IO"=w1057:errorcluster)  [unwired: 7 in]
      }
      frame "UpdateSubClassKernels" {
        n475 = Unbundle By Name(w1136) -> ("Classes"=w1149:T2[])
        n476 = for {
          tunnel: w1149 -> [w1153] mode=indexing
          tunnel: [w1152] -> w1148 mode=indexing
          tunnel: [w1151] -> w1140 mode=indexing
          n477 = Unbundle By Name(w1153) -> ("ClassName"=w1152:string, "ClassFolder"=w1151:path)
        }
        n478 = Format Into String(EndevoTemplateNames."BaseTemplate" ("TemplateNames")) -> (resulting string=w1144:string)  [unwired: 3 in, 1 out]
        n479 = call <resource>:"GOOP300_GetClassTemplatePath.vi"("ClassTemplateSubDirectory"=w1144) -> ("FolderPathOut"=w1145:path)  [unwired: 17 in, 1 out]
        n480 = Build Path(base path=w1145, name or relative path="utils") -> (appended path=w1143:path)
        n481 = Build Path(base path=w1143, name or relative path="BaseTemplate_GOOPKernel.vi") -> (appended path=w1141:path)
        n482 = for {
          tunnel: w1149 -> [w1175] mode=indexing
          shift-right: [w1162] -> w1138
          shift-left: w1150 -> [w1163]
          tunnel: w1148 -> [w1161]
          tunnel: w1141 -> [w1160]
          tunnel: w1140 -> [w1159]
          n483 = Unbundle By Name(w1175) -> ("InheritsFrom"=w1164:path, "ClassName"=w1157:string, "ViRefs"=w1169:refnum<vi>[], "ViPathes"=w1173:path[])
          n484 = for {
            tunnel: w1173 -> [w1180] mode=indexing
            tunnel: "GOOPKernel.vi$" ("regular expression") -> [w1178]
            tunnel: [w1176] -> w1171 mode=indexing
            n485 = Strip Path(path=w1180) -> (name=w1179:string)  [unwired: 1 out]
            n486 = Match Pattern(string=w1179, regular expression=w1178) -> (offset past match=w1177:i32)  [unwired: 1 in, 3 out]
            n487 = Greater Or Equal To 0?(x=w1177) -> (x >= 0?=w1176:bool)
          }
          n488 = Strip Path(path=w1164) -> (name=w1165:string)  [unwired: 1 out]
          n489 = Match Pattern(string=w1165, regular expression="_[Cc][Ll][Aa][Ss][Ss]") -> (before substring=w1156:string)  [unwired: 1 in, 3 out]
          n490 = Empty String/Path?(string/path=w1164) -> (empty?=w1174:bool)
          n491 = Match Pattern(string=w1156, regular expression="[.][Ll][Ll][Bb]$") -> (before substring=w1154:string)  [unwired: 1 in, 3 out]
          n492 = Search 1D Array(1D array=w1171, element=TRUE) -> (index of element=w1168:i32)  [unwired: 1 in]
          n493 = Index Array(array=w1169, index=w1168) -> (element=w1167:refnum<vi>)
          n494 = Search 1D Array(1D array=w1161, element=w1154) -> (index of element=w1158:i32)  [unwired: 1 in]
          n495 = case shown="False" w1174 {
            tunnel: w1167 -> [w1201 _]
            tunnel: w1163 -> [w1181 w1203]
            tunnel: [w1181 w1203] -> w1162
            tunnel: w1160 -> [w1200 _]
            tunnel: w1159 -> [w1198 _]
            tunnel: w1158 -> [w1197 _]
            tunnel: w1157 -> [w1192 _]
            frame False {
              n496 = Index Array(array=w1198, index=w1197) -> (element=w1196:path)
              n497 = call <vilib>:"Recursive File List.vi"("pattern"="*GOOPKernel.vi", "Treat LLBs as Folders?"=TRUE, "Folder Path"=w1196) -> ("All Files in Dir"=w1193:path[])  [unwired: 4 in, 4 out]
              n498 = Build Array(w1200) -> (w1199:path[])
              n499 = Format Into String(format string="Updating kernel: %s", w1192) -> (resulting string=w1182:string)  [unwired: 2 in, 1 out]
              n500 = call <resource>:"Scripting_ReplaceVisAndControls.vi"("ViRef"=w1201, "OldVIsAndControls"=w1199, "NewVIsAndControls"=w1193, "error in (no error)"=w1181) -> ()  [unwired: 14 in, 2 out]
              n501 = property on="Progress" class="LstBox (strict)"() -> ("Item Names"=w1190:string[], "Number of Rows"=w1184:u32)  [unwired: 2 in, 2 out]
              n502 = Build Array (concatenate)(w1190, w1182) -> (w1185:string[])
              n503 = stacked-sequence {
                tunnel: w1181 -> [_]
                frame #0 {
                  n504 = Wait (ms)(milliseconds to wait=u32 5) -> ()  [unwired: 1 out]
                }
              }
              n505 = Array Size(array=w1185) -> (size(s)=w1189:i32)
              n506 = Subtract(x=w1189, y=w1184) -> (x-y=w1188:u32)
              n507 = To Long Integer(number=w1188) -> (32bit integer=w1186:i32)
              n508 = Max & Min(x=w1186, y=0) -> (max(x,y)=w1183:i32)  [unwired: 1 out]
              n509 = property on="Progress" class="LstBox (strict)"("Item Names"=w1185, "Top Row"=w1183) -> ()  [unwired: 2 in, 2 out]
            }
            frame True {
            }
          }
        }
        n510 = call <resource>:"ConvertGoop2ToGoop3_RecompileAll.vi"("error IO 2"=w1138, "Cluster 2"=w1136) -> ("error IO"=w1137:errorcluster)  [unwired: 7 in]
      }
      frame "UpdateVIsGoopRefs" {
        n511 = Unbundle By Name(w1204) -> ("Classes"=w1211:T2[])
        n512 = for {
          tunnel: w1211 -> [w1225] mode=indexing
          tunnel: [w1223] -> w1207 mode=indexing
          n513 = Unbundle By Name(w1225) -> ("ClassRef"=w1224:refnum<vi>)
          n514 = property class="LVClassLibrary"(reference=w1224) -> ("Path"=w1223:path)  [unwired: 1 in, 2 out]
        }
        n515 = for {
          tunnel: w1211 -> [w1242] mode=indexing
          shift-right: [w1226] -> w1209
          shift-left: w1212 -> [w1241]
          tunnel: w1207 -> [w1239]
          n516 = Unbundle By Name(w1242) -> ("ViRefs"=w1240:refnum<vi>[], "ViPathes"=w1238:path[], "ClassName"=w1228:string)  [unwired: 2 out]
          n517 = for {
            shift-right: [w1256] -> w1226
            shift-left: w1241 -> [w1257]
            tunnel: w1240 -> [w1247] mode=indexing
            tunnel: w1239 -> [w1255]
            tunnel: w1238 -> [w1249] mode=indexing
            tunnel: [w1248] -> _
            n518 = Strip Path(path=w1249) -> (stripped path=w1254:path, name=w1251:string)
            n519 = Path To String(path=w1249) -> (string=w1248:string)
            n520 = Match Pattern(string=w1251, regular expression="\\2E[Vv][Ii]$") -> ()  [unwired: 1 in, 4 out]
            n521 = Strip Path(path=w1254) -> (name=w1253:string)  [unwired: 1 out]
            n522 = Not Equal?(x=w1253, y="utils") -> (x != y?=w1246:bool)
            n523 = Not A Number/Path/Refnum?(number/path/refnum=w1247) -> (NaN/Path/Refnum?=w1245:bool)
            n524 = Compound Arithmetic op=AND(invert w1245, w1246) -> (w1244:bool)
            n525 = case shown="True" w1244 {
              tunnel: w1257 -> [w1258 w1259]
              tunnel: [w1258 w1259] -> w1256
              tunnel: w1247 -> [_ w1261]
              tunnel: w1255 -> [_ w1260]
              frame False {
              }
              frame True {
                n526 = call <resource>:"Scripting_ReplaceGoop2OORef.vi"("ViRef"=w1261, "Classes(.lvclass files)"=w1260, "error in (no error)"=w1259) -> ()  [unwired: 16 in, 1 out]
              }
            }
          }
          n527 = Format Into String(format string="Updating GOOP Ref: %s", w1228) -> (resulting string=w1227:string)  [unwired: 2 in, 1 out]
          n528 = property on="Progress" class="LstBox (strict)"() -> ("Item Names"=w1237:string[], "Number of Rows"=w1231:u32)  [unwired: 2 in, 2 out]
          n529 = Build Array (concatenate)(w1237, w1227) -> (w1232:string[])
          n530 = Array Size(array=w1232) -> (size(s)=w1236:i32)
          n531 = Subtract(x=w1236, y=w1231) -> (x-y=w1235:u32)
          n532 = To Long Integer(number=w1235) -> (32bit integer=w1233:i32)
          n533 = Max & Min(x=w1233, y=0) -> (max(x,y)=w1230:i32)  [unwired: 1 out]
          n534 = property on="Progress" class="LstBox (strict)"("Item Names"=w1232, "Top Row"=w1230) -> ()  [unwired: 2 in, 2 out]
          n535 = stacked-sequence {
            tunnel: w1226 -> [_]
            frame #0 {
              n536 = Wait (ms)(milliseconds to wait=u32 5) -> ()  [unwired: 1 out]
            }
          }
        }
        n537 = Unbundle By Name(w1204) -> ("VIsToRelink"=w1208:refnum<vi>[])
        n538 = for {
          shift-right: [w1213] -> w1206
          shift-left: w1209 -> [w1217]
          tunnel: w1208 -> [w1216] mode=indexing
          tunnel: w1207 -> [w1214]
          n539 = Not A Number/Path/Refnum?(number/path/refnum=w1216) -> (NaN/Path/Refnum?=w1215:bool)
          n540 = case shown="False" w1215 {
            tunnel: w1217 -> [w1221 w1222]
            tunnel: [w1221 w1222] -> w1213
            tunnel: w1216 -> [w1220 _]
            tunnel: w1214 -> [w1219 _]
            frame False {
              n541 = call <resource>:"Scripting_ReplaceGoop2OORef.vi"("ViRef"=w1220, "Classes(.lvclass files)"=w1219, "error in (no error)"=w1221) -> ()  [unwired: 16 in, 1 out]
            }
            frame True {
            }
          }
          n542 = stacked-sequence {
            tunnel: w1213 -> [_]
            frame #0 {
              n543 = Wait (ms)(milliseconds to wait=u32 5) -> ()  [unwired: 1 out]
            }
          }
        }
        n544 = call <resource>:"ConvertGoop2ToGoop3_RecompileAll.vi"("error IO 2"=w1206, "Cluster 2"=w1204) -> ("error IO"=w1205:errorcluster)  [unwired: 7 in]
      }
      frame "UpdateCreate" {
        n545 = Unbundle By Name(w1263) -> ("Classes"=w1268:T2[])
        n546 = for {
          tunnel: w1268 -> [w1294] mode=indexing
          shift-right: [w1282] -> w1267
          shift-left: w1269 -> [w1296]
          tunnel: [w1298] -> w1265 mode=indexing
          n547 = Unbundle By Name(w1294) -> ("ViRefs"=w1297:refnum<vi>[], "ClassName"=w1283:string)
          n548 = for {
            tunnel: w1297 -> [w1307] mode=indexing
            shift-right: [w1308] -> w1295
            shift-left: w1296 -> [w1309]
            n549 = call <resource>:"Scripting_SaveVi.vi"("error in (no error)"=w1309, "VIRefToSaveIn"=w1307) -> ("error out"=w1308:errorcluster)  [unwired: 8 in, 1 out]
          }
          n550 = Unbundle By Name(w1294) -> ("ViRefs"=w1301:refnum<vi>[], "ViPathes"=w1305:path[])  [unwired: 2 out]
          n551 = Format Into String(format string="Updating Create: %s", w1283) -> (resulting string=w1284:string)  [unwired: 2 in, 1 out]
          n552 = for {
            tunnel: w1305 -> [w1318] mode=indexing
            tunnel: "_Create.vi$" ("regular expression") -> [w1316]
            tunnel: [w1314] -> w1303 mode=indexing
            n553 = Strip Path(path=w1318) -> (name=w1317:string)  [unwired: 1 out]
            n554 = Match Pattern(string=w1317, regular expression=w1316) -> (offset past match=w1315:i32)  [unwired: 1 in, 3 out]
            n555 = Greater Or Equal To 0?(x=w1315) -> (x >= 0?=w1314:bool)
          }
          n556 = property on="Progress" class="LstBox (strict)"() -> ("Item Names"=w1293:string[], "Number of Rows"=w1287:u32)  [unwired: 2 in, 2 out]
          n557 = Build Array (concatenate)(w1293, w1284) -> (w1288:string[])
          n558 = Array Size(array=w1288) -> (size(s)=w1292:i32)
          n559 = Subtract(x=w1292, y=w1287) -> (x-y=w1291:u32)
          n560 = To Long Integer(number=w1291) -> (32bit integer=w1289:i32)
          n561 = Search 1D Array(1D array=w1303, element=TRUE) -> (index of element=w1300:i32)  [unwired: 1 in]
          n562 = Index Array(array=w1301, index=w1300) -> (element=w1299:refnum<vi>)
          n563 = Max & Min(x=w1289, y=0) -> (max(x,y)=w1286:i32)  [unwired: 1 out]
          n564 = property on="Progress" class="LstBox (strict)"("Item Names"=w1288, "Top Row"=w1286) -> ()  [unwired: 2 in, 2 out]
          n565 = case shown="0, Default" w1300 {
            tunnel: w1295 -> [w1310 w1313]
            tunnel: [w1310 w1313] -> w1282
            tunnel: w1299 -> [w1312 _]
            tunnel: [w1312 _] -> w1298
            frame 0, Default {
              n566 = call <resource>:"Scripting_UpdateGoop2Create.vi"("ViRef"=w1312, "RemovePreloadDynamicMethods"=FALSE, "error in (no error)"=w1310) -> ()  [unwired: 16 in, 1 out]
            }
            frame -1 {
            }
          }
          n567 = stacked-sequence {
            tunnel: w1282 -> [_]
            frame #0 {
              n568 = Wait (ms)(milliseconds to wait=u32 5) -> ()  [unwired: 1 out]
            }
          }
        }
        n569 = Unbundle By Name(w1263) -> ("AppRef"=w1262:refnum<vi>)
        n570 = for {
          shift-right: [w1273] -> w1266
          shift-left: w1267 -> [w1274]
          tunnel: w1265 -> [w1272] mode=indexing
          tunnel: w1262 -> [w1270]
          n571 = Not A Number/Path/Refnum?(number/path/refnum=w1272) -> (NaN/Path/Refnum?=w1271:bool)
          n572 = case shown="False" w1271 {
            tunnel: path "PreloadDynamicMethods.vi" ("Path") -> [w1280 _]
            tunnel: w1274 -> [w1277 w1281]
            tunnel: [w1277 w1281] -> w1273
            tunnel: w1272 -> [w1279 _]
            tunnel: w1270 -> [w1276 _]
            frame False {
              n573 = call <resource>:"Scripting_RemoveSubViAndFixWires.vi"("MainViPath/ViRef/BlockDiagramRef"=w1279, "SubVIToRemove"=w1280, "SaveVIBeforeRemove(False)"=TRUE, "error in (no error)"=w1277, "AppRef"=w1276) -> ()  [unwired: 14 in, 1 out]
            }
            frame True {
            }
          }
        }
      }
      frame "UpdateDynamicDispatchVIs" {
        n574 = call <resource>:"ConvertGoop2ToGoop3_RecompileAll.vi"("error IO 2"=w1321, "Cluster 2"=w1319) -> ("error IO"=w1320:errorcluster)  [unwired: 7 in]
        n575 = Unbundle By Name(w1319) -> ("Classes"=w1326:T2[])
        n576 = for {
          tunnel: w1326 -> [w1330] mode=indexing
          shift-right: [w1328] -> w1327
          shift-left: w1320 -> [w1350]
          tunnel: w1326 -> [w1347]
          shift-right: [w1341] -> w1323
          shift-left: refnum<vi>[] [] -> [w1342]
          i -> [w1346]
          n577 = Unbundle By Name(w1330) -> ("ClassName"=w1329:string)
          n578 = Delete From Array(array=w1347, index=w1346) -> (array with subset deleted=w1345:T2[])  [unwired: 1 in, 1 out]
          n579 = for {
            tunnel: w1345 -> [w1356] mode=indexing
            shift-right: [w1354] -> w1343
            shift-left: string[] [] -> [w1355]
            n580 = Unbundle By Name(w1356) -> ("ViPathes"=w1352:path[])
            n581 = for {
              tunnel: [w1358] -> w1353 mode=indexing
              tunnel: w1352 -> [w1357] mode=indexing
              n582 = Strip Path(path=w1357) -> (name=w1358:string)  [unwired: 1 out]
            }
            n583 = Build Array (concatenate)(w1355, w1353) -> (w1354:string[])
          }
          n584 = Unbundle By Name(w1330) -> ("ViRefs"=w1349:refnum<vi>[], "ViPathes"=w1348:path[])  [unwired: 2 out]
          n585 = Format Into String(format string="Updating dynamic dispatch: %s", w1329) -> (resulting string=w1332:string)  [unwired: 2 in, 1 out]
          n586 = property on="Progress" class="LstBox (strict)"() -> ("Item Names"=w1340:string[], "Number of Rows"=w1334:u32)  [unwired: 2 in, 2 out]
          n587 = Build Array (concatenate)(w1340, w1332) -> (w1335:string[])
          n588 = for {
            shift-right: [w1375] -> w1328
            shift-left: w1350 -> [w1376]
            tunnel: w1349 -> [w1361] mode=indexing
            tunnel: w1348 -> [w1374] mode=indexing
            tunnel: w1343 -> [w1368]
            shift-right: [w1364] -> w1341
            shift-left: w1342 -> [w1363]
            n589 = Strip Path(path=w1374) -> (stripped path=w1373:path, name=w1370:string)
            n590 = To Lower Case(string=w1368) -> (all lower case string=w1367:string[])
            n591 = To Lower Case(string=w1370) -> (all lower case string=w1369:string)
            n592 = Strip Path(path=w1373) -> (name=w1362:string)  [unwired: 1 out]
            n593 = Search 1D Array(1D array=w1367, element=w1369) -> (index of element=w1366:i32)  [unwired: 1 in]
            n594 = Not Equal?(x=w1362, y="utils") -> (x != y?=w1371:bool)
            n595 = Not A Number/Path/Refnum?(number/path/refnum=w1361) -> (NaN/Path/Refnum?=w1359:bool)
            n596 = Greater Or Equal To 0?(x=w1366) -> (x >= 0?=w1365:bool)
            n597 = Compound Arithmetic op=AND(invert w1359, w1371) -> (w1360:bool)
            n598 = case shown="True" w1360 {
              tunnel: w1376 -> [w1378 w1383]
              tunnel: [w1378 w1383] -> w1375
              tunnel: w1361 -> [_ w1380]
              tunnel: w1365 -> [_ w1384]
              tunnel: [w1377 w1382] -> w1364
              tunnel: w1363 -> [w1377 w1381]
              frame False {
              }
              frame True {
                n599 = call <resource>:"Scripting_RemoveDynamicDispatchInGoop2VIs.vi"("ViRef"=w1380, "ForceDynamicDispatch"=w1384, "error in (no error)"=w1383) -> ("DynamicDispatch"=w1379:bool)  [unwired: 15 in, 1 out]
                n600 = case shown="True" w1379 {
                  tunnel: [w1385 w1388] -> w1382
                  tunnel: w1381 -> [w1385 w1387]
                  tunnel: w1380 -> [_ w1386]
                  frame False {
                  }
                  frame True {
                    n601 = Build Array (concatenate)(w1387, w1386) -> (w1388:refnum<vi>[])
                  }
                }
              }
            }
          }
          n602 = Array Size(array=w1335) -> (size(s)=w1339:i32)
          n603 = Subtract(x=w1339, y=w1334) -> (x-y=w1338:u32)
          n604 = To Long Integer(number=w1338) -> (32bit integer=w1336:i32)
          n605 = Max & Min(x=w1336, y=0) -> (max(x,y)=w1333:i32)  [unwired: 1 out]
          n606 = property on="Progress" class="LstBox (strict)"("Item Names"=w1335, "Top Row"=w1333) -> ()  [unwired: 2 in, 2 out]
          n607 = stacked-sequence {
            tunnel: w1328 -> [_]
            frame #0 {
              n608 = Wait (ms)(milliseconds to wait=u32 5) -> ()  [unwired: 1 out]
            }
          }
        }
        n609 = Bundle By Name(cluster=w1319, "SetToDynamicDispatch"=w1323) -> (w1324:T7)
      }
      frame "ExtraSave" {
        n610 = call <resource>:"ConvertGoop2ToGoop3_RecompileAll.vi"("error IO 2"=w1401, "Cluster 2"=w1399) -> ("error IO"=w1400:errorcluster)  [unwired: 7 in]
        n611 = property on="Progress" class="LstBox (strict)"() -> ("Item Names"=w1398:string[], "Number of Rows"=w1392:u32)  [unwired: 2 in, 2 out]
        n612 = Build Array (concatenate)(w1398, "Recompiling VIs again") -> (w1393:string[])
        n613 = Array Size(array=w1393) -> (size(s)=w1397:i32)
        n614 = Subtract(x=w1397, y=w1392) -> (x-y=w1396:u32)
        n615 = To Long Integer(number=w1396) -> (32bit integer=w1394:i32)
        n616 = Max & Min(x=w1394, y=0) -> (max(x,y)=w1391:i32)  [unwired: 1 out]
        n617 = property on="Progress" class="LstBox (strict)"("Item Names"=w1393, "Top Row"=w1391) -> ()  [unwired: 2 in, 2 out]
      }
      frame "SetDynamicDispatch" {
        n618 = Unbundle By Name(w1414) -> ("SetToDynamicDispatch"=w1402:refnum<vi>[])
        n619 = property on="Progress" class="LstBox (strict)"() -> ("Item Names"=w1412:string[], "Number of Rows"=w1406:u32)  [unwired: 2 in, 2 out]
        n620 = Build Array (concatenate)(w1412, "Setting dynamic dispatch" ("format string")) -> (w1407:string[])
        n621 = Array Size(array=w1407) -> (size(s)=w1411:i32)
        n622 = Subtract(x=w1411, y=w1406) -> (x-y=w1410:u32)
        n623 = To Long Integer(number=w1410) -> (32bit integer=w1408:i32)
        n624 = Max & Min(x=w1408, y=0) -> (max(x,y)=w1405:i32)  [unwired: 1 out]
        n625 = property on="Progress" class="LstBox (strict)"("Item Names"=w1407, "Top Row"=w1405) -> (error out=w1403:errorcluster)  [unwired: 2 in, 1 out]
        n626 = for {
          N -> [w1417]
          tunnel: w1402 -> [w1420] mode=indexing
          tunnel: w1403 -> [_]
          i -> [w1418]
          n627 = Not A Number/Path/Refnum?(number/path/refnum=w1420) -> (NaN/Path/Refnum?=w1419:bool)
          n628 = Increment(x=w1418) -> (x+1=w1416:i32)
          n629 = case shown="False" w1419 {
            tunnel: w1420 -> [w1425 _]
            tunnel: w1416 -> [w1422 _]
            tunnel: w1417 -> [w1421 _]
            frame False {
              n630 = property class="VI"(reference=w1425) -> (error out=w1433:errorcluster, "ConPane"=w1431:refnum<vi>, "Path"=w1430:path)  [unwired: 1 in, 1 out]
              n631 = Strip Path(path=w1430) -> (stripped path=w1429:path, name=w1424:string)
              n632 = stacked-sequence {
                tunnel: w1424 -> [w1434]
                tunnel: [w1434] -> w1423
                frame #0 {
                  w1438 = path "c:/G2To3.txt" ("file (use dialog)")
                  n633 = Read from Text File(file (use dialog)=w1438) -> (text=w1435:string)  [unwired: 3 in, 3 out]
                  n634 = Concatenate Strings(w1435, w1434, "\n" ("string")) -> (w1436:string)
                  n635 = stacked-sequence {
                    tunnel: w1436 -> [w1441]
                    tunnel: w1438 -> [w1439]
                    frame #0 {
                      n636 = Delete(path (use dialog)=w1439) -> (deleted path=w1440:path)  [unwired: 4 in, 2 out]
                      n637 = Write to Text File(file (use dialog)=w1440, text=w1441) -> ()  [unwired: 2 in, 3 out]
                    }
                  }
                }
              }
              n638 = Strip Path(path=w1429) -> (name=w1427:string)  [unwired: 1 out]
              n639 = Not Equal?(x=w1427, y="private") -> (x != y?=w1426:bool)
              n640 = case shown="True" w1426 {
                tunnel: w1433 -> [_ w1461]
                tunnel: [w1442 w1460] -> w1432
                tunnel: w1431 -> [w1442 w1458]
                tunnel: w1423 -> [_ w1447]
                tunnel: w1422 -> [_ w1445]
                tunnel: w1421 -> [_ w1444]
                frame False {
                }
                frame True {
                  w1459 = T14."Dynamic Dispatch" ("Rule")
                  n641 = Not Equal?(x="Destroy.vi", y=w1447) -> ()  [unwired: 1 out]
                  n642 = Format Into String(format string="Setting dynamic dispatch: %d of %d (%s)", w1445, w1444, w1447) -> (resulting string=w1452:string)  [unwired: 2 in, 1 out]
                  n643 = invoke class="ConPane" method="SetWireRule"(reference=w1458, error in=w1461, "TermIdx"=u32 0 ("Terminal Index"), "Rule"=w1459) -> (reference out=w1455:refnum<vi>, error out=w1456:errorcluster)  [unwired: 1 in, 3 out]
                  n644 = property on="Progress" class="LstBox (strict)" props=["Item Names", "Number of Rows"]() -> ("Item Names"=w1451:string[])  [unwired: 2 in, 3 out]
                  n645 = Array Size(array=w1451) -> (size(s)=w1450:i32)
                  n646 = Decrement(x=w1450) -> (x-1=w1449:i32)
                  n647 = Replace Array Subset(array=w1451, new element=w1452, index=w1449) -> (w1454:string[])
                  n648 = case shown="True" TRUE {
                    tunnel: [w1463 w1469] -> w1460
                    tunnel: w1459 -> [_ w1468]
                    tunnel: w1456 -> [w1462 w1466]
                    tunnel: w1455 -> [w1463 w1465]
                    tunnel: [w1462 w1464] -> w1448
                    frame False {
                    }
                    frame True {
                      n649 = invoke class="ConPane" method="SetWireRule"(reference=w1465, error in=w1466, "TermIdx"=u32 14 ("Terminal Index"), "Rule"=w1468) -> (reference out=w1469:refnum<vi>, error out=w1464:errorcluster)  [unwired: 1 in, 3 out]
                    }
                  }
                  n650 = property on="Progress" class="LstBox (strict)"("Item Names"=w1454) -> ()  [unwired: 2 in, 2 out]
                  n651 = stacked-sequence {
                    tunnel: w1448 -> [_]
                    frame #0 {
                      n652 = Wait (ms)(milliseconds to wait=u32 5) -> ()  [unwired: 1 out]
                    }
                  }
                }
              }
              n653 = Close Reference(reference=w1432) -> ()  [unwired: 1 in, 1 out]
            }
            frame True {
            }
          }
        }
      }
      frame "UpdateAllCallParentMethods" {
        n654 = Unbundle By Name(w1471) -> ("CallParentMethod"=w1475:cluster{"VIRef":refnum<vi>, "Position":T6}[])
        n655 = call <resource>:"ConvertGoop2ToGoop3_RecompileAll.vi"("error IO 2"=w1473, "Cluster 2"=w1471) -> ("error IO"=w1472:errorcluster)  [unwired: 7 in]
        n656 = for {
          tunnel: w1475 -> [w1496] mode=indexing
          shift-right: [w1482] -> w1474
          shift-left: w1472 -> [w1490]
          w1484 = 2354 items=[".NET Container"=2125, ".NET Refnum"=3441, "3D Picture Control"=23776, "Absolute Value"=1054, "Access Rights"=1412, "ActiveX Container"=2072, "Add"=3915, "Add 1"=1050, "Add Array Elements"=1903, "Agitator"=3831, "AllSpoll"=1960, "Always Copy"=2400, "And"=1061, "And Array Elements"=1911, "Append True/False String"=1511, "Application Refnum"=3412, "Array"=21608, "Array 1"=3300, "Array Constant"=2070, "Array Max & Min"=1907, "Array Size"=1809, "Array Subset"=2044, "Array To Cluster"=1168, "Array To Spreadsheet String"=1540, "Array of Strings to Path"=1422, "Atmospheric Tank"=21751, "Atmospheric Tank 1"=3070, "Automation Close"=8001, "Automation Open"=8000, "Automation Refnum"=3410, "Avogadro Constant (1/mol)"=23520, "Base 10 Logarithm Of e"=23512, "Bin"=21755, "Bin 1"=3073, "Bluetooth Close Connection"=9148, "Bluetooth Create Listener"=9151, "Bluetooth Discover"=9152, "Bluetooth Network Connection Refnum"=3468, "Bluetooth Open Connection"=9153, "Bluetooth Read"=9149, "Bluetooth Wait On Listener"=9147, "Bluetooth Write"=9150, "Boolean Array To Number"=1815, "Boolean To (0,1)"=1167, "Build Array"=2041, "Build Cluster Array"=2047, "Build Path"=1419, "Build Waveform"=2066, "Bundle"=2049, "Bundle By Name"=2057, "Byte Array To String"=1609, "Byte Stream File Refnum"=3408, "CAN Channel"=21966, "CAN Channel 1"=3340, "CAN Channel 2"=2124, "CAN Channel 3"=21817, "CAN Interface"=3339, "CAN Interface 1"=21815, "CAN Interface 2"=2123, "CAN Interface 3"=21964, "CAN Task"=3470, "CAN Task 1"=3471, "CAN Task 2"=21963, "CAN Task 3"=21789, "Call By Reference Node"=3901, "Call Chain"=1999, "Call Library Function Node"=2062, "Call Parent Method"=2354, "Cancel Button"=21739, "Cancel Notification"=9107, "Carriage Return Constant"=23500, "Case Structure"=2001, "Cast Unit Bases"=1079, "Check Valve"=3833, "Checkbox"=3117, "Class Specifier Constant"=2094, "Classic Radio Buttons"=22003, "Close File"=8052, "Close File 1"=1405, "Close Reference"=8011, "Cluster"=21607, "Cluster 1"=3400, "Cluster Constant"=2071, "Cluster To Array"=1169, "Code Interface Node"=2050, "Coerce To Type"=2402, "Color Box"=3013, "Color Box Constant"=2120, "Color Box Thin Border"=2905, "Color Ramp"=3022, "Combo Box"=3304, "Combo Box 1"=21604, "Combo Box Constant"=2088, "Complex Conjugate"=1048, "Complex To Polar"=1045, "Complex To Re/Im"=1044, "Compound Arithmetic"=2200, "Compressor"=3832, "Concatenate Strings"=2040, "Conditional Disable Structure"=2064, "Constructor Node"=3904, "Control Help Window"=1353, "Control Online Help"=1355, "Control Refnum"=3419, "Convert Unit"=2059, "Conveyer"=3827, "Copy"=8053, "Copy 1"=1416, "Cosecant"=1204, "Cosine"=1201, "Cotangent"=1205, "Create Folder"=8055, "Create User Event"=2073, "Current VI's Menubar"=9000, "Current VI's Path"=1426, "DAQmx Analog Trigger Source"=21774, "DAQmx Analog Trigger Source 1"=3336, "DAQmx Analog Trigger Source 2"=2119, "DAQmx Analog Trigger Source 3"=21951, "DAQmx Device Name"=3318, "DAQmx Device Name 1"=21773, "DAQmx Device Name 2"=21950, "DAQmx Device Name 3"=2093, "DAQmx Global Channel"=3430, "DAQmx Global Channel 1"=3443, "DAQmx Global Channel 2"=21770, "DAQmx Global Channel 3"=21957, "DAQmx Physical Channel"=21777, "DAQmx Physical Channel 1"=3335, "DAQmx Physical Channel 2"=21954, "DAQmx Physical Channel 3"=2118, "DAQmx Scale Name"=2116, "DAQmx Scale Name 1"=21952, "DAQmx Scale Name 2"=21775, "DAQmx Scale Name 3"=3317, "DAQmx Switch"=21776, "DAQmx Switch 1"=21953, "DAQmx Switch 2"=3337, "DAQmx Switch 3"=2121, "DAQmx Task Name"=21778, "DAQmx Task Name 1"=3442, "DAQmx Task Name 2"=3434, "DAQmx Task Name 3"=21959, "DAQmx Terminal"=3319, "DAQmx Terminal 1"=21955, "DAQmx Terminal 2"=2117, "DAQmx Terminal 3"=21781, "Data Log File Refnum"=3402, "DataSocket Close"=1085, "DataSocket Open"=1084, "DataSocket Read"=1086, "DataSocket Refnum"=3417, "DataSocket Write"=1087, "Date/Time To Seconds"=1308, "Decimal Digit?"=1119, "Decimal String To Number"=1184, "Decimate 1D Array"=2046, "Decrement"=1058, "Default Directory"=1427, "Delete"=1417, "Delete 1"=8056, "Delete From Array"=3912, "Delete Menu Items"=9004, "Delete Variant Attribute"=8206, "Delete Waveform Attribute"=8209, "Deny Access"=8057, "Dequeue Element"=9113, "Destroy User Event"=2075, "DevClear"=1961, "DevClearList"=1962, "Device Control/Status"=1433, "Device Refnum"=3405, "Diagram Disable Structure"=2054, "Dial"=3050, "Dial 1"=21732, "Digital Data"=3210, "Digital Data 1"=21216, "Digital Waveform Graph"=3502, "Digital Waveform Graph 1"=21718, "Digital Waveform Graph 2"=3511, "Divide"=3918, "Divide 1"=1053, "Dlg CheckBox"=21924, "Dlg Horiz Scrollbar"=21905, "Dlg Numeric"=2100, "Dlg Numeric 2"=3006, "Dlg String"=2110, "Dlg Vert Scrollbar"=21906, "Down Arrow"=3824, "Down Bow Valve"=3807, "Down Bow Valve 1"=21767, "Down Bow Valve 2"=3707, "Down Rect Valve"=21766, "Down Rect Valve 1"=3806, "Down Rect Valve 2"=3706, "Down Tee"=3718, "Down Tee 1"=3818, "EOF"=1410, "Elementary Charge (C)"=23517, "Empty Array?"=23063, "Empty Path Constant"=23523, "Empty String Constant"=23503, "Empty String/Path?"=1112, "Empty Variant"=8200, "Enable Menu Tracking"=9002, "EnableLocal"=1963, "EnableRemote"=1964, "End of Line Constant"=23525, "Enqueue Element"=9111, "Enqueue Element At Opposite End"=9129, "Enum"=3023, "Enum 1"=21605, "Enum Constant"=2090, "Equal To 0?"=1113, "Equal?"=1102, "Error Ring Constant"=2039, "Event Callback Refnum"=3435, "Event Data Node"=2102, "Event Structure"=2052, "Exchanger"=3828, "Exclusive Or"=1063, "Exponential"=1211, "Exponential (Arg) -1"=1222, "Expression Node"=2201, "False Constant"=2006, "Feedback Node"=2353, "FieldPoint IO Point"=3440, "FieldPoint IO Point 1"=21784, "FieldPoint IO Point 2"=3439, "File Dialog"=8081, "File Dialog 1"=8058, "File Path Control"=3203, "File Path Control 1"=21730, "File Path Indicator"=3204, "File Path Indicator 1"=21731, "File/Directory Info"=8082, "File/Directory Info 1"=1413, "FindLstn"=1965, "FindRQS"=1966, "First Call?"=1083, "Flat Box"=3602, "Flat Circle"=3605, "Flat Down Triangle"=3623, "Flat Frame"=3608, "Flat Left Triangle"=3620, "Flat Right Triangle"=3621, "Flat Round Button"=3102, "Flat Rounded Box"=3611, "Flat Sequence Structure"=2069, "Flat Square Button"=3103, "Flat Up Triangle"=3622, "Flatten To String"=1164, "Flatten To XML"=8400, "Flattened String To Variant"=8202, "Floating Point Equal?"=23064, "Flush File"=1406, "Flush File 1"=8059, "Flush Queue"=9114, "For Loop"=2002, "Format Date/Time String"=8100, "Format Into File"=2083, "Format Into String"=2081, "Format Value"=1512, "Formula Node"=2004, "Fract/Exp String To Number"=1187, "Framed Color Box"=21019, "Framed Color Box 1"=3008, "Free Label"=2321, "Furnace"=3829, "GPIB Clear"=1954, "GPIB Initialization"=1957, "GPIB Misc"=1956, "GPIB Read"=1951, "GPIB Serial Poll"=1955, "GPIB Status"=1959, "GPIB Trigger"=1953, "GPIB Wait"=1958, "GPIB Write"=1950, "Gauge"=21009, "Gauge 1"=3040, "Generate Front Panel Activity"=1329, "Generate Occurrence"=1700, "Generate User Event"=2074, "Get Datalog Position"=8061, "Get Date/Time In Seconds"=1303, "Get Date/Time String"=1600, "Get Drag Drop Data"=9154, "Get File Position"=8062, "Get File Size"=8063, "Get Help Window Status"=1354, "Get Menu Item Info"=9005, "Get Menu Selection"=9001, "Get Menu Short Cut Info"=9007, "Get Notifier Status"=9103, "Get Number of Records"=8064, "Get Permissions"=8065, "Get Queue Status"=9110, "Get Type and Creator"=8066, "Get Variant Attribute"=8205, "Get Volume Info"=8067, "Get Waveform Attribute"=8208, "Get Waveform Components"=2067, "Global Variable"=2060, "Gravitational Constant (N m2/kg2)"=23519, "Greater Or Equal To 0?"=1114, "Greater Or Equal?"=1103, "Greater Than 0?"=1117, "Greater?"=1110, "Handle Peek"=1604, "Handle Poke"=1605, "Hex Digit?"=1123, "Hexadecimal String To Number"=1185, "Hopper"=3072, "Hopper 1"=21754, "Horiz Line"=3821, "Horiz Pipe"=3710, "Horiz Pipe 1"=3810, "Horizontal Button Box"=3636, "Horizontal Fill Slide"=21100, "Horizontal Fill Slide 1"=3012, "Horizontal Graduated Bar"=21106, "Horizontal Pointer Slide"=3011, "Horizontal Pointer Slide 1"=21101, "Horizontal Progress Bar"=21102, "Horizontal Scrollbar"=21110, "Horizontal Slide"=3010, "Horizontal Slide Switch"=3114, "Horizontal Smooth Box"=3633, "Horizontal Splitter Bar"=21861, "Horizontal Splitter Bar (Classic)"=21863, "Horizontal Splitter Bar (System)"=21865, "Horizontal Switch"=3108, "Horizontal Tank"=3071, "Horizontal Toggle Switch"=21700, "Horizontal Toggle Switch 1"=3110, "Hyperbolic Cosecant"=23053, "Hyperbolic Cosine"=1215, "Hyperbolic Cotangent"=23055, "Hyperbolic Secant"=23054, "Hyperbolic Sine"=1214, "Hyperbolic Tangent"=1216, "IMAQ Session"=3415, "IP To String"=1710, "IVI Delete Session"=8103, "IVI Logical Name"=3414, "IVI Logical Name 1"=21736, "IVI Logical Name 2"=3420, "IVI New Session"=8102, "Implies"=1080, "In Range and Coerce"=1127, "Increment"=1057, "Index & Bundle Cluster Array"=2056, "Index Array"=2042, "Index String Array"=1531, "Initialize Array"=2053, "Inline C Node"=2104, "Input"=1351, "Insert Into Array"=3911, "Insert Menu Items"=9003, "Intensity Chart"=3509, "Intensity Chart 1"=21719, "Intensity Graph"=3510, "Intensity Graph 1"=21720, "Interleave 1D Arrays"=2045, "Interpolate 1D Array"=1905, "Inverse Cosecant"=23050, "Inverse Cosine"=1207, "Inverse Cotangent"=23052, "Inverse Hyperbolic Cosecant"=23056, "Inverse Hyperbolic Cosine"=1218, "Inverse Hyperbolic Cotangent"=23058, "Inverse Hyperbolic Secant"=23057, "Inverse Hyperbolic Sine"=1217, "Inverse Hyperbolic Tangent"=1219, "Inverse Secant"=23051, "Inverse Sine"=1206, "Inverse Tangent"=1208, "Inverse Tangent (2 Input)"=1228, "Invoke Node"=3900, "IrDA Close Connection"=9144, "IrDA Create Listener"=9140, "IrDA Discover"=9141, "IrDA Network Connection Refnum"=3450, "IrDA Open Connection"=9142, "IrDA Read"=9145, "IrDA Wait On Listener"=9143, "IrDA Write"=9146, "Join Numbers"=1171, "Knob"=3005, "Knob 1"=21000, "LED Button"=3116, "LabVIEW Object"=3457, "Label"=21960, "Labeled Oblong Button"=3125, "Labeled Rectangular Button"=3124, "Labeled Round Button"=3122, "Labeled Square Button"=3123, "Left Arrow"=3826, "Left Bow Valve"=3801, "Left Bow Valve 1"=3701, "Left Bow Valve 2"=21761, "Left Down Elbow"=3711, "Left Down Elbow 1"=3811, "Left Pump"=3713, "Left Pump 1"=3813, "Left Rect Valve"=3800, "Left Rect Valve 1"=21760, "Left Rect Valve 2"=3700, "Left Tee"=3709, "Left Tee 1"=3809, "Left Up Elbow"=3808, "Left Up Elbow 1"=3708, "Less Or Equal To 0?"=1115, "Less Or Equal?"=1104, "Less Than 0?"=1118, "Less?"=1111, "Lexical Class"=1126, "Line Feed Constant"=23501, "List Directory"=1418, "List Folder"=8083, "Listbox"=21806, "Listbox 1"=21792, "Listbox Symbol Ring Constant"=2038, "Local Variable"=2061, "Lock Range"=1411, "Logarithm Base 10"=1210, "Logarithm Base 2"=1225, "Logarithm Base X"=1224, "Logical Shift"=1081, "Lookup Table Refnum"=3426, "Lowered Rounded Box"=3638, "MATLAB Script Node"=9020, "Machine Epsilon"=23528, "MakeAddr"=1967, "Mantissa & Exponent"=1150, "Match First String"=1532, "Match Pattern"=1535, "Match True/False String"=1533, "MathScript Node"=2357, "Max & Min"=1108, "Menu Refnum"=3413, "Menu Ring"=3018, "Menu Ring 1"=21600, "Menu-Popup Ring"=3017, "Merge Signals"=2350, "Meter"=21008, "Meter 1"=3030, "Mixed Signal Graph"=21721, "Molar Gas Constant (J/(mol K))"=23522, "Motion Resource"=3449, "Motion Resource 1"=21787, "Motion Resource 2"=3448, "Motor"=3820, "Motor 1"=3720, "Move"=1415, "Move 1"=8068, "Multicolumn Listbox"=21791, "Multicolumn Listbox 1"=21799, "Multiple Selection Listbox"=3208, "Multiply"=3917, "Multiply 1"=1052, "Multiply Array Elements"=1904, "Multirate Structure"=2199, "Natural Logarithm"=1209, "Natural Logarithm (Arg +1)"=1221, "Natural Logarithm Base"=23510, "Natural Logarithm Of 10"=23513, "Natural Logarithm Of 2"=23514, "Natural Logarithm Of Pi"=23508, "Negate"=1069, "Negative Infinity"=23509, "New Directory"=1402, "New File"=1404, "New VI"=8014, "New VI Object"=8015, "Not"=1064, "Not A Number/Path/Refnum?"=1128, "Not A Path Constant"=23524, "Not And"=1071, "Not Equal To 0?"=1116, "Not Equal?"=1105, "Not Exclusive Or"=1073, "Not Or"=1072, "Not a Refnum Constant"=23526, "Not a Shared Variable"=23527, "Notifier Refnum"=3423, "Number To Boolean Array"=1814, "Number To Decimal String"=1180, "Number To Engineering String"=1183, "Number To Exponential String"=1505, "Number To Fractional String"=1506, "Number To Hexadecimal String"=1181, "Number To Octal String"=1182, "Numeric Constant"=2005, "Numeric Control"=3000, "Numeric Control 1"=21003, "Numeric Indicator"=3001, "Numeric Indicator 1"=21004, "OK Button"=21738, "OLE Variant"=3150, "Obtain Notifier"=9101, "Obtain Queue"=9108, "Occurrence Refnum"=3406, "Octal Digit?"=1129, "Octal String To Number"=1186, "Old VISA Open"=1921, "One Button Dialog"=1340, "Open Application Reference"=8012, "Open Device"=1430, "Open File"=1403, "Open Tank"=21752, "Open Tank 1"=3074, "Open VI Object Reference"=8013, "Open VI Reference"=8010, "Open/Create/Replace Datalog"=8054, "Open/Create/Replace File"=8050, "Or"=1062, "Or Array Elements"=1910, "PPoll"=1969, "PPollConfig"=1970, "PPollUnconfig"=1971, "Package Matrix"=23001, "PassControl"=1968, "Path Constant"=2009, "Path To String"=1077, "Path Type"=1421, "Path to Array of Strings"=1423, "Pi"=23504, "Pi Divided By 2"=23506, "Pi Multiplied By 2"=23505, "Pick Line"=1510, "Pict Ring"=3015, "Pict Ring 1"=21602, "Picture"=3508, "PixMap"=3505, "PixMap (Do not touch it!!)"=3507, "Planck Constant (J/Hz)"=23516, "Platform Flat Square Button"=3134, "Plug-In Control"=21820, "Polar To Complex"=1047, "Polar To Re/Im"=23061, "Positive Infinity"=23515, "Power Of 10"=1212, "Power Of 2"=1223, "Power Of X"=1213, "Pressure Tank"=21753, "Pressure Tank 1"=3075, "Preview Queue Element"=9112, "Printable?"=1124, "Priority Queue Refnum"=3425, "Property Node"=1920, "Pulldown Menu Ring"=3061, "Push Button"=21001, "Queue Refnum"=3474, "Queue Refnum 1"=3424, "Quit LabVIEW"=1352, "Quotient & Remainder"=1056, "RT FIFO Create"=24000, "RT FIFO Delete"=24003, "RT FIFO Read"=24001, "RT FIFO Write"=24002, "Radio Buttons"=22001, "Raised Box"=3637, "Raised Box 1"=3600, "Raised Circle"=3603, "Raised Down Triangle"=3615, "Raised Frame"=3606, "Raised Left Triangle"=3612, "Raised Right Triangle"=3613, "Raised Rounded Box"=3609, "Raised Up Triangle"=3614, "Random Number (0-1)"=1070, "RcvRespMsg"=1972, "Re/Im To Complex"=1046, "Re/Im To Polar"=23060, "Read Datalog"=8069, "Read Device"=1432, "Read File"=1407, "Read from Binary File"=8051, "Read from Text File"=8070, "ReadStatus"=1973, "Receive"=1974, "ReceiveSetup"=1975, "Recessed Box"=3601, "Recessed Circle"=3604, "Recessed Down Triangle"=3619, "Recessed Frame"=3607, "Recessed Left Triangle"=3616, "Recessed Menu Ring"=3019, "Recessed Right Triangle"=3617, "Recessed Rounded Box"=3610, "Recessed Up Triangle"=3618, "Reciprocal"=1059, "Reciprocal Of Pi"=23507, "Reciprocal Of e"=23511, "Rectangular Stop Button"=3128, "Refnum to Path"=1424, "Refnum to Session"=2306, "Register Event Callback"=2078, "Register For Events"=2065, "Register Session"=2319, "Release Notifier"=9102, "Release Queue"=9109, "Replace Array Subset"=3910, "Replace Substring"=3913, "Request Deallocation"=1610, "ResetSys"=1976, "Reshape Array"=2055, "Reverse 1D Array"=1900, "Reverse String"=1537, "Right Arrow"=3825, "Right Bow Valve"=21765, "Right Bow Valve 1"=3805, "Right Bow Valve 2"=3705, "Right Down Elbow"=3717, "Right Down Elbow 1"=3817, "Right Pump"=3819, "Right Pump 1"=3719, "Right Rect Valve"=3704, "Right Rect Valve 1"=3804, "Right Rect Valve 2"=21764, "Right Tee"=3815, "Right Tee 1"=3715, "Right Up Elbow"=3714, "Right Up Elbow 1"=3814, "Ring Constant"=2008, "Rocker"=21002, "Rotary Feeder"=3830, "Rotate"=1082, "Rotate 1D Array"=1906, "Rotate Left With Carry"=1606, "Rotate Right With Carry"=1607, "Rotate String"=1536, "Round Button"=3100, "Round LED"=3120, "Round LED 1"=21012, "Round Light"=3104, "Round Push Button"=3112, "Round Push Button 2"=3118, "Round Radio Button"=3106, "Round Stop Button"=3127, "Round To +Infinity"=1076, "Round To -Infinity"=1075, "Round To Nearest"=1055, "Rydberg Constant (1/m)"=23521, "Scale By Power Of 2"=1074, "Scan From File"=2082, "Scan From String"=2080, "Scan String For Tokens"=8101, "Scan Value"=1534, "Search 1D Array"=1901, "Search and Replace String"=3914, "Search/Split String"=1538, "Secant"=1203, "Seconds To Date/Time"=1309, "Seek"=1409, "Select"=1516, "Send"=1977, "Send Notification"=9104, "SendCmds"=1978, "SendDataBytes"=1979, "SendIFC"=1980, "SendLLO"=1982, "SendList"=1981, "SendSetup"=1983, "Session to Refnum"=2307, "Set Datalog Position"=8072, "Set File Position"=8073, "Set File Size"=8074, "Set Menu Item Info"=9006, "Set Number of Records"=8075, "Set Occurrence"=1702, "Set Permissions"=8076, "Set Type and Creator"=8077, "Set Variant Attribute"=8204, "Set Waveform Attribute"=8207, "SetRWLS"=1984, "SetTimeOut"=1985, "Shared Variable Constant"=3473, "Shared Variable Control"=21814, "Shared Variable Control 1"=3472, "Shared Variable to String"=1831, "Sign"=1049, "Simple Horizontal Slide"=3003, "Simple Numeric"=3029, "Simple Numeric 1"=2900, "Simple String"=2115, "Simple Vertical Slide"=3002, "Simulation Loop"=2099, "Sinc"=1227, "Sine"=1200, "Sine & Cosine"=1220, "Size Handle"=1603, "Slide Switch"=21011, "Sort 1D Array"=1120, "Sort Array of String, Sort Array of String 1"=23065, "Speed Of Light In Vacuum (m/sec)"=23518, "Split 1D Array"=1908, "Split Button"=21020, "Split Number"=1170, "Split Signals"=2351, "Spreadsheet String To Array"=1539, "Square"=23059, "Square Button"=3101, "Square LED"=3121, "Square LED 1"=21013, "Square Light"=3105, "Square Push Button"=3113, "Square Push Button 2"=3119, "Square Radio Button"=3107, "Square Root"=1060, "Stacked Sequence Structure"=2000, "State Diagram"=2051, "Static VI Reference"=2084, "Stop"=1350, "Stop Button"=21230, "String Constant"=2007, "String Control"=21701, "String Control 1"=3200, "String Indicator"=21702, "String Indicator 1"=3201, "String Length"=1502, "String Subset"=1503, "String To Byte Array"=1608, "String To IP"=1711, "String To Path"=1078, "String to Shared Variable"=1830, "Strip Path"=1420, "SubPanel"=21810, "SubPanel (Classic)"=21811, "Subtract"=3916, "Subtract 1"=1051, "Swap Bytes"=1162, "Swap Values"=2401, "Swap Vector Element"=1912, "Swap Words"=1163, "System Button"=3130, "System Cancel Button"=3131, "System Checkbox"=3132, "System Chiseled Line"=3632, "System Colored Rectangle"=3625, "System Combo Box"=21917, "System Enum"=3062, "System Horizontal Pointer Slide"=21902, "System Horizontal Progress Bar"=21910, "System Horizontal Slide"=21904, "System Label"=21961, "System Listbox"=21805, "System Multicolumn Listbox"=21798, "System Numeric"=21919, "System Path Control"=21922, "System Pict Ring"=21925, "System Radio Button"=3133, "System Radio Buttons"=22002, "System Recessed Frame"=3624, "System Ring"=3060, "System Spin Control"=21900, "System String"=21920, "System Tab Control"=3331, "System Table"=21797, "System Time Stamp"=21967, "System Tree"=21794, "System Vertical Pointer Slide"=21901, "System Vertical Progress Bar"=21909, "System Vertical Slide"=21903, "TCP Close Connection"=1713, "TCP Create Listener"=1717, "TCP Flattened Read"=1718, "TCP Flattened Write"=1719, "TCP Flex Read"=1720, "TCP Flex Write"=1721, "TCP Network Connection Refnum"=3407, "TCP Open Connection"=1715, "TCP Read"=1716, "TCP Wait On Listener"=1712, "TCP Write"=1714, "TDMS Close"=2013, "TDMS Defragment"=2019, "TDMS File"=3477, "TDMS Flush"=2017, "TDMS Get Properties"=2015, "TDMS List Contents"=2016, "TDMS Open"=2012, "TDMS Read"=2011, "TDMS Set Properties"=2014, "TDMS Write"=2010, "TDMS Write IP"=2018, "Tab Constant"=23502, "Tab Control"=3332, "Tab Control 1"=3330, "Table"=21796, "Table 1"=21790, "Tag Attribute Ring"=2063, "Tag Constant"=2089, "Tag Control"=3302, "Tag Control 1"=21742, "Tag Indicator"=3303, "Tag Indicator 1"=21743, "Tangent"=1202, "Tank"=21006, "Tank 1"=3020, "Temporary Directory"=1435, "TestSRQ"=1986, "TestSys"=1987, "Text & Pict Ring"=21603, "Text & Pict Ring 1"=3016, "Text Button"=21015, "Text Ring"=21601, "Text Ring 1"=3014, "Text to UTF-8"=23066, "Thermometer"=21007, "Thermometer 1"=3021, "Thick Chiseled Line"=3630, "Thick Line"=3629, "Thick Line with Arrow"=3631, "Thick Lowered Box"=3635, "Thin Chiseled Line"=3627, "Thin Line"=3626, "Thin Line with Arrow"=3628, "Threshold 1D Array"=1909, "Tick Count (ms)"=1300, "Time Stamp Constant"=2068, "Time Stamp Control"=5555, "Time Stamp Control 1"=21913, "Time Stamp Indicator"=5556, "Time Stamp Indicator 1"=21914, "Timed Loop"=5570, "Timed Sequence"=5573, "To Byte Integer"=1140, "To Double Precision Complex"=1152, "To Double Precision Float"=1147, "To Extended Precision Complex"=1154, "To Extended Precision Float"=1149, "To Long Integer"=1142, "To Lower Case"=1189, "To More Generic Class"=8017, "To More Specific Class"=8016, "To OLE Variant"=8002, "To Quad Integer"=1155, "To Single Precision Complex"=1151, "To Single Precision Float"=1146, "To Time Stamp"=5560, "To Unsigned Byte Integer"=1143, "To Unsigned Long Integer"=1145, "To Unsigned Quad Integer"=1156, "To Unsigned Word Integer"=1144, "To Upper Case"=1188, "To Variant"=8201, "To Word Integer"=1141, "Traditional DAQ Channel"=21733, "Traditional DAQ Channel 1"=3320, "Traditional DAQ Channel 2"=2085, "Transpose 2D Array"=1902, "Tree"=21819, "Tree 1"=21793, "Trigger"=1988, "TriggerList"=1989, "Two Button Dialog"=1341, "Type Cast"=1166, "Type and Creator"=1434, "UDP Close"=1726, "UDP Multicast Open"=1727, "UDP Network Connection Refnum"=3418, "UDP Open"=1723, "UDP Read"=1724, "UDP Write"=1725, "UTF-8 to Text"=23067, "Unbundle"=2048, "Unbundle By Name"=2058, "Unflatten From String"=1165, "Unflatten From XML"=8401, "Unpackage Matrix"=23000, "Unregister For Events"=2076, "Unregister Session"=2320, "Up Arrow"=3823, "Up Bow Valve"=21763, "Up Bow Valve 1"=3803, "Up Bow Valve 2"=3703, "Up Rect Valve"=3702, "Up Rect Valve 1"=3802, "Up Rect Valve 2"=21762, "Up Tee"=3712, "Up Tee 1"=3812, "User Defined Refnum"=3428, "User Defined Refnum Tag"=3429, "User Defined Refnum Tag 1"=21745, "User Defined Refnum Tag Flatten"=3454, "User Defined Refnum Tag Flatten 1"=21747, "User Defined Tag"=2114, "User Defined Tag 1"=21749, "User Item"=3506, "VI Library"=1425, "VI Refnum"=3422, "VI Server Reference"=2091, "VISA Assert Interrupt Signal"=2309, "VISA Assert Trigger"=1929, "VISA Assert Utility Signal"=2310, "VISA Clear"=1927, "VISA Close"=1922, "VISA Disable Event"=1940, "VISA Discard Events"=1941, "VISA Enable Event"=1942, "VISA Find Resource"=1923, "VISA Flush I/O Buffer"=2302, "VISA GPIB Command"=2315, "VISA GPIB Control ATN"=2316, "VISA GPIB Control REN"=2304, "VISA GPIB Pass Control"=2317, "VISA GPIB Send IFC"=2318, "VISA In 16"=1930, "VISA In 32"=1944, "VISA In 8"=1936, "VISA Lock"=1993, "VISA Map Address"=1932, "VISA Map Trigger"=2311, "VISA Memory Allocation"=1997, "VISA Memory Free"=1998, "VISA Move"=2303, "VISA Move In 16"=1948, "VISA Move In 32"=1991, "VISA Move In 8"=1946, "VISA Move Out 16"=1949, "VISA Move Out 32"=1992, "VISA Move Out 8"=1947, "VISA Open"=2308, "VISA Out 16"=1931, "VISA Out 32"=1945, "VISA Out 8"=1937, "VISA Peek 16"=1934, "VISA Peek 32"=1995, "VISA Peek 8"=1938, "VISA Poke 16"=1935, "VISA Poke 32"=1996, "VISA Poke 8"=1939, "VISA Read"=1925, "VISA Read STB"=1928, "VISA Read To File"=2313, "VISA Refnum to Session"=2300, "VISA Resource Name"=21737, "VISA Resource Name 1"=3421, "VISA Set I/O Buffer Size"=2301, "VISA Status Description"=1924, "VISA USB Control In"=2086, "VISA USB Control Out"=2087, "VISA Unlock"=1994, "VISA Unmap Address"=1933, "VISA Unmap Trigger"=2312, "VISA VXI Cmd or Query"=2305, "VISA Wait on Event"=1943, "VISA Write"=1926, "VISA Write From File"=2314, "VISA resource name"=3409, "Variant"=3310, "Variant To Data"=8003, "Variant To Flattened String"=8203, "Vert Line"=3822, "Vert Pipe"=3716, "Vert Pipe 1"=3816, "Vert Rocker"=21740, "Vertical Fill Slide"=21014, "Vertical Fill Slide 1"=3009, "Vertical Graduated Bar"=21107, "Vertical Pointer Slide"=21017, "Vertical Pointer Slide 1"=3007, "Vertical Progress Bar"=21104, "Vertical Scrollbar"=21111, "Vertical Slide"=3004, "Vertical Slide Switch"=21741, "Vertical Slide Switch 1"=3115, "Vertical Smooth Box"=3634, "Vertical Splitter Bar"=21860, "Vertical Splitter Bar (Classic)"=21862, "Vertical Splitter Bar (System)"=21864, "Vertical Switch"=3109, "Vertical Toggle Switch"=21005, "Vertical Toggle Switch 1"=3111, "Volume Info"=1414, "Wait (ms)"=1302, "Wait For Activity"=1722, "Wait For Front Panel Activity"=1328, "Wait Until Next ms Multiple"=1327, "Wait for GPIB RQS"=1952, "Wait on Notification"=9105, "Wait on Notification from Multiple"=9106, "Wait on Occurrence"=1701, "WaitSRQ"=1990, "Waveform Chart"=3501, "Waveform Chart 1"=21717, "Waveform Chart 2"=21010, "Waveform Graph"=21703, "Waveform Graph 1"=3504, "While Loop"=2003, "While Loop 1"=2352, "White Space?"=1125, "Write Datalog"=8079, "Write Device"=1431, "Write File"=1408, "Write to Binary File"=8078, "Write to Text File"=8080, "XY Graph"=3500, "XY Graph 1"=21716, "Xmath Script Node"=9022, "Y-th root of X"=23062] ("ExchangeType")
          w1488 = refnum<vi> refnum  # Node
          n657 = Unbundle By Name(w1496) -> ("VIRef"=w1481:refnum<vi>, "Position"=w1477:T6)
          n658 = property class="VI"(reference=w1481) -> ("Path"=w1480:path)  [unwired: 1 in, 2 out]
          n659 = Build Array (concatenate)(path[] [path "Unknown", path ""] ("VIsToSerachFor"), w1480) -> (w1478:path[])
          n660 = call <resource>:"Scripting_FindVisOnDiagram.vi"("ViRef"=w1481, "VIsToSerachFor/ViName"=w1478, "error in (no error)"=w1490) -> ("VisFound"=w1495:refnum<vi>[], "error out"=w1491:errorcluster)  [unwired: 15 in]
          n661 = for {
            tunnel: w1495 -> [w1501] mode=indexing
            tunnel: [w1500] -> w1494 mode=indexing
            tunnel: [w1499] -> w1493 mode=indexing
            shift-right: [w1498] -> w1485
            shift-left: w1491 -> [w1497]
            n662 = property class="GObj"(reference=w1501, error in=w1497) -> (reference out=w1499:refnum<vi>, error out=w1498:errorcluster, "Position"=w1500:T6)
          }
          n663 = Search 1D Array(1D array=w1494, element=w1477) -> (index of element=w1492:i32)  [unwired: 1 in]
          n664 = Index Array(array=w1493, index=w1492) -> (element=w1489:refnum<vi>)
          n665 = To More Specific Class(target class=w1488, reference=w1489, error in=w1485) -> (specific class reference=w1487:refnum<vi>, error out=w1486:errorcluster)
          n666 = call <resource>:"Scripting_ExchangeNodeAndRewire.vi"("Node"=w1487, "ExchangeType"=w1484, "error in (no error)"=w1486) -> ("error out"=w1483:errorcluster)  [unwired: 16 in]
          n667 = call <vilib>:"Clear Errors.vi"("error in (no error)"=w1483) -> ("error out"=w1482:errorcluster)  [unwired: 5 in, 1 out]
        }
      }
      frame "UpdateDestroy" {
        n668 = Unbundle By Name(w1506) -> ("Classes"=w1505:T2[])
        n669 = for {
          tunnel: w1505 -> [w1510] mode=indexing
          shift-right: [w1508] -> w1503
          shift-left: w1507 -> [w1528]
          n670 = Unbundle By Name(w1510) -> ("ViRefs"=w1523:refnum<vi>[], "ViPathes"=w1527:path[])  [unwired: 2 out]
          n671 = Unbundle By Name(w1510) -> ("ClassName"=w1509:string)
          n672 = for {
            tunnel: w1527 -> [w1538] mode=indexing
            tunnel: "destroy.vi$" ("regular expression") -> [w1536]
            tunnel: [w1534] -> w1525 mode=indexing
            n673 = Strip Path(path=w1538) -> (name=w1537:string)  [unwired: 1 out]
            n674 = To Lower Case(string=w1537) -> (all lower case string=w1533:string)
            n675 = Match Pattern(string=w1533, regular expression=w1536) -> (offset past match=w1535:i32)  [unwired: 1 in, 3 out]
            n676 = Greater Or Equal To 0?(x=w1535) -> (x >= 0?=w1534:bool)
          }
          n677 = Search 1D Array(1D array=w1525, element=TRUE) -> (index of element=w1522:i32)  [unwired: 1 in]
          n678 = Index Array(array=w1523, index=w1522) -> (element=w1521:refnum<vi>)
          n679 = case shown="0, Default" w1522 {
            tunnel: w1528 -> [w1530 w1532]
            tunnel: [w1530 w1532] -> w1508
            tunnel: w1521 -> [w1531 _]
            frame 0, Default {
              n680 = call <resource>:"Scripting_UpdateGoop2Destroy.vi"("ViRef"=w1531, "error in (no error)"=w1530) -> ()  [unwired: 17 in, 1 out]
            }
            frame -1 {
            }
          }
          n681 = Format Into String(format string="Update destory methods: %s", w1509) -> (resulting string=w1512:string)  [unwired: 2 in, 1 out]
          n682 = property on="Progress" class="LstBox (strict)"() -> ("Item Names"=w1520:string[], "Number of Rows"=w1514:u32)  [unwired: 2 in, 2 out]
          n683 = Build Array (concatenate)(w1520, w1512) -> (w1515:string[])
          n684 = Array Size(array=w1515) -> (size(s)=w1519:i32)
          n685 = Subtract(x=w1519, y=w1514) -> (x-y=w1518:u32)
          n686 = To Long Integer(number=w1518) -> (32bit integer=w1516:i32)
          n687 = stacked-sequence {
            tunnel: w1508 -> [_]
            frame #0 {
              n688 = Wait (ms)(milliseconds to wait=u32 5) -> ()  [unwired: 1 out]
            }
          }
          n689 = Max & Min(x=w1516, y=0) -> (max(x,y)=w1513:i32)  [unwired: 1 out]
          n690 = property on="Progress" class="LstBox (strict)"("Item Names"=w1515, "Top Row"=w1513) -> ()  [unwired: 2 in, 2 out]
        }
        n691 = call <resource>:"ConvertGoop2ToGoop3_RecompileAll.vi"("error IO 2"=w1503) -> ("error IO"=w1502:errorcluster)  [unwired: 8 in]
      }
      frame "UpdateClassInfo" {
        n692 = Unbundle By Name(w1550) -> ("Classes"=w1552:T2[])
        n693 = for {
          tunnel: w1552 -> [w1559] mode=indexing
          shift-right: [w1555] -> w1539
          shift-left: w1551 -> [w1564]
          n694 = Unbundle By Name(w1559) -> ("ClassRef"=w1557:refnum<vi>, "TemplateVersionUsed"=w1556:string)
          n695 = Unbundle By Name(w1559) -> ("InheritsFrom"=w1563:path)
          n696 = property class="LVClassLibrary"(reference=w1557, error in=w1564) -> (reference out=w1571:refnum<vi>, error out=w1572:errorcluster, "Description"=w1570:string)
          n697 = Empty String/Path?(string/path=w1563) -> (empty?=w1562:bool)
          n698 = Select(t=EndevoTemplateNames."BaseTemplate" ("TemplateNames"), s=w1562, f=EndevoTemplateNames."SubTemplate" ("TemplateNames")) -> (s? t:f=w1558:T10)
          n699 = Format Into String(w1558) -> (resulting string=w1569:string)  [unwired: 3 in, 1 out]
          n700 = Format Into String(EndevoProviderName."EndevoGOOP300" ("ProviderName")) -> (resulting string=w1568:string)  [unwired: 3 in, 1 out]
          n701 = Bundle By Name(cluster=T3 {"ClassProviderName"="", "ClassTemplateUsed"="", "ClassTemplateVersion"="", "ClassDescription"="", "PlugIns"=[], "ConnectorPanePattern"=""} ("ClassSettings"), "ClassProviderName"=w1568, "ClassTemplateUsed"=w1569, "ClassTemplateVersion"=w1556, "ClassDescription"=w1570) -> (w1566:T3)
          n702 = call <resource>:"GDSLvClass_StoreClassType.vi"("Class Refnum In"=w1571, "ClassSettings"=w1566, "error in (no error)"=w1572) -> ("Class Refnum Out"=w1553:refnum<vi>, "error out"=w1554:errorcluster)  [unwired: 15 in]
          n703 = invoke class="LVClassLibrary" method="Save"(reference=w1553, error in=w1554) -> ()  [unwired: 2 in, 4 out]
          n704 = stacked-sequence {
            tunnel: w1554 -> [_]
            frame #0 {
              n705 = Wait (ms)(milliseconds to wait=u32 5) -> ()  [unwired: 1 out]
            }
          }
          n706 = call <vilib>:"Clear Errors.vi"("error in (no error)"=w1554) -> ("error out"=w1555:errorcluster)  [unwired: 5 in, 1 out]
        }
        n707 = property on="Progress" class="LstBox (strict)"() -> ("Item Names"=w1548:string[], "Number of Rows"=w1542:u32)  [unwired: 2 in, 2 out]
        n708 = Build Array (concatenate)(w1548, "Update class info") -> (w1543:string[])
        n709 = Array Size(array=w1543) -> (size(s)=w1547:i32)
        n710 = Subtract(x=w1547, y=w1542) -> (x-y=w1546:u32)
        n711 = To Long Integer(number=w1546) -> (32bit integer=w1544:i32)
        n712 = Max & Min(x=w1544, y=0) -> (max(x,y)=w1541:i32)  [unwired: 1 out]
        n713 = property on="Progress" class="LstBox (strict)"("Item Names"=w1543, "Top Row"=w1541) -> ()  [unwired: 2 in, 2 out]
      }
    }
    n714 = call <vilib>:"Clear Errors.vi"("error in (no error)"=w19) -> ("error out"=w18:errorcluster)  [unwired: 5 in, 1 out]
    n715 = Equal?(x=w29, y="Exit") -> (x = y?=w32:bool)
    n716 = Select(t="Error", s=w18, f=w29) -> (s? t:f=w33:string)
    "State" <- w23
  }
  n717 = Unbundle By Name(w13) -> ("error"=w10:errorcluster)
  n718 = call <resource>:"GDSError_ReportError.vi"("error in (no error)"=w10) -> ("error out"=w1:errorcluster)  [unwired: 18 in]
  "error out" <- w1
  n719 = property class="VI"(reference=w4, error in=w1, "Front Panel.Open"=FALSE ("Front Panel Window:Open")) -> (reference out=w2:refnum<vi>, error out=w3:errorcluster)
  n720 = Close Reference(reference=w2, error in (no error)=w3) -> ()  [unwired: 1 out]
